vi "LDLTS measurement.vi"(5 "Session properties":T5, 7 "Workspace":path, 8 "Error In":errorcluster, 9 "myDLTS file path":path=path "", 10 "LDLTS measurement":T2={"Name"="", "Comment"="", "Time"=timestamp(0 s since 1904-01-01), "Folder"=path "", "LDLTS properties"={"T"=0.0, "Test signal"=0.0, "Test frequency"=0.0, "Bandwidth"=0.0, "Averaging"=0.0, "Vbias"=0.0, "Vpulse"=0.0, "pulse length"=0.0, "Pulse 2"=FALSE, "Vpulse 2"=0.0, "pulse length 2"=0.0, "I range"=-2.0, "V range"=10.0, "Sampling rate"=0.0, "Acq. delay"=0.0, "Sampling time"=0.0, "Filter order"=0, "Equivalent circuit model"=0}, "GUID"=""} {"LDLTS properties"."Equivalent circuit model" items=["Rp || Cp", "Rs + Cs", "Rs + Ls", "G B", "D Cs", "Q Cs", "D Ls", "Q Ls", "Rp || Lp", "D Cp"]; "LDLTS properties"."Filter order" min=0 max=8 step=1; "LDLTS properties"."Sampling rate" items=["13k"=13392.857422, "27k"=26785.714844, "54k"=53571.429687, "107k"=107142.859375]; "LDLTS properties"."V range" items=["10mV"=0.01, "100mV"=0.1, "1V"=1.0, "10V"=10.0]; "LDLTS properties"."I range" items=["100nA"=-7.0, "1µA"=-6.0, "10µA"=-5.0, "100µA"=-4.0, "1mA"=-3.0, "10mA"=-2.0]}, 11 "Loop data":T6={"Persistent"={"Last file"=path "", "Last user"="", "Users"=[]}, "Temp handle"={"Connected"=FALSE, "Temp ctrl"={"Gain (P)"=0.0, "Reset (I)"=0.0, "Rate (D)"=0.0, "Stabilization rate"=0.0, "Stabilization delta"=0.0, "Type"=enum."Lake Shore 325", "Custom temp ctrl"={"VISA resource name"=""}, "Lakeshore 325"={"VISA name"="", "Loop"=0, "Heater Range"=1, "Heater Resistance"=0, "Sample sensor"=0, "Fast sensor"=0, "Slow sensor"=0}, "Lakeshore 331"={"VISA name"="", "Loop"=1, "Heater Range"=0, "Sample sensor"=0, "Fast sensor"=0, "Slow sensor"=0}, "Lakeshore 332"={"VISA name"="", "Loop"=1, "Heater Range"=0, "Sample sensor"=0, "Fast sensor"=0, "Slow sensor"=0}, "Lakeshore 335"={"VISA name"="", "Loop"=1, "Sample sensor"=0, "Fast sensor"=0, "Slow sensor"=0, "Heater Range"=0, "Output mode"=enum."Off"}, "Lakeshore 336"={"VISA name"="", "Loop"=1, "Output mode"=enum."Off", "Max current"=1.0, "Heater resistance"=1, "Sample sensor"=1, "Slow sensor"=1, "Fast sensor"=1}}}, "Paths"={"Manual"=path "", "Settings"=path "", "Persistent"=path "", "Work dir."=path ""}, "Settings"={"MFIA"={"Address"="", "Use compensation"=TRUE, "Shut down gracefully"=FALSE}, "Temp ctrl"={"Gain (P)"=0.0, "Reset (I)"=0.0, "Rate (D)"=0.0, "Stabilization rate"=0.0, "Stabilization delta"=0.0, "Type"=enum."Lake Shore 325", "Custom temp ctrl"={"VISA resource name"=""}, "Lakeshore 325"={"VISA name"="", "Loop"=0, "Heater Range"=1, "Heater Resistance"=0, "Sample sensor"=0, "Fast sensor"=0, "Slow sensor"=0}, "Lakeshore 331"={"VISA name"="", "Loop"=1, "Heater Range"=0, "Sample sensor"=0, "Fast sensor"=0, "Slow sensor"=0}, "Lakeshore 332"={"VISA name"="", "Loop"=1, "Heater Range"=0, "Sample sensor"=0, "Fast sensor"=0, "Slow sensor"=0}, "Lakeshore 335"={"VISA name"="", "Loop"=1, "Sample sensor"=0, "Fast sensor"=0, "Slow sensor"=0, "Heater Range"=0, "Output mode"=enum."Off"}, "Lakeshore 336"={"VISA name"="", "Loop"=1, "Output mode"=enum."Off", "Max current"=1.0, "Heater resistance"=1, "Sample sensor"=1, "Slow sensor"=1, "Fast sensor"=1}}, "Source-meter"={"Type"=enum."Custom", "Custom source-meter"={"VISA resource name"=""}, "Keithley 2600"={"VISA name"="", "Ignore ID Query"=FALSE, "SMU"=enum."Channel A"}, "Keithley 2400 Series"={"VISA name"="", "Ignore ID Query"=FALSE}}, "Other"={"Enable OriginLab"=FALSE, "Reader mode"=FALSE, "Auto-save"=FALSE}, "Defaults"={"IV properties"={"T"=0.0, "Vstart"=-0.5, "Vstop"=0.5, "Vpoints"=10.0, "Settling"=0.01, "I limit"=0.1, "Log mapping"=FALSE, "Averaging"=0.0}, "CV properties"={"T"=0.0, "Vstart"=-0.5, "Vstop"=0.5, "Vpoints"=10.0, "Precision"=enum."Normal", "Test signal"=0.01, "Auto I range"=FALSE, "Test frequency"=100000.0, "I range"=-2.0, "V range"=10.0, "Log mapping"=FALSE, "Rel perm"=0.0, "Area"=0.0, "Equivalent circuit model"=0}, "DLTS properties"={"Tstart"=0.0, "Instant start"=FALSE, "Tstop"=0.0, "T rate"=0.0, "Test signal"=0.0, "Test frequency"=0.0, "Bandwidth"=0.0, "Averaging"=0.0, "Vbias"=0.0, "Vpulse"=0.0, "pulse length"=0.0, "Pulse 2"=FALSE, "Vpulse 2"=0.0, "pulse length 2"=0.0, "I range"=-2.0, "V range"=10.0, "Emission rate"=[], "Sampling rate"=0.0, "Acq. delay"=0.0, "Filter order"=0, "Equivalent circuit model"=0}, "LDLTS properties"={"T"=0.0, "Test signal"=0.0, "Test frequency"=0.0, "Bandwidth"=0.0, "Averaging"=0.0, "Vbias"=0.0, "Vpulse"=0.0, "pulse length"=0.0, "Pulse 2"=FALSE, "Vpulse 2"=0.0, "pulse length 2"=0.0, "I range"=-2.0, "V range"=10.0, "Sampling rate"=0.0, "Acq. delay"=0.0, "Sampling time"=0.0, "Filter order"=0, "Equivalent circuit model"=0}}}, "Software version"=0.0, "MFIA handle"={"ziHandle"={"handleValid"=FALSE, "Conn"=0, "Path Prefix"="", "Handle"=0, "Connected"=FALSE, "Clockbase(s)"=0.0}, "Selected device"="", "ziModHandle"={"handleValid"=FALSE, "Conn"=0, "ModHandle"=0, "moduleID"="", "Path Prefix"=""}}, "Source-meter handle"={"Connected"=FALSE, "Source-meter"={"Type"=enum."Custom", "Custom source-meter"={"VISA resource name"=""}, "Keithley 2600"={"VISA name"="", "Ignore ID Query"=FALSE, "SMU"=enum."Channel A"}, "Keithley 2400 Series"={"VISA name"="", "Ignore ID Query"=FALSE}}}} {"MFIA handle"."ziModHandle"."ModHandle" format="0x%08x"; "MFIA handle"."ziModHandle"."Conn" format="0x%08x"; "MFIA handle"."ziHandle"."Handle" format="0x%08x"; "MFIA handle"."ziHandle"."Conn" format="0x%08x"; "Settings"."Defaults"."LDLTS properties"."Equivalent circuit model" items=["Rp || Cp", "Rs + Cs", "Rs + Ls", "G B", "D Cs", "Q Cs", "D Ls", "Q Ls", "Rp || Lp", "D Cp"]; "Settings"."Defaults"."LDLTS properties"."Filter order" min=0 max=8 step=1; "Settings"."Defaults"."LDLTS properties"."Sampling rate" items=["13k"=13392.857422, "27k"=26785.714844, "54k"=53571.429687, "107k"=107142.859375]; "Settings"."Defaults"."LDLTS properties"."V range" items=["10mV"=0.01, "100mV"=0.1, "1V"=1.0, "10V"=10.0]; "Settings"."Defaults"."LDLTS properties"."I range" items=["100nA"=-7.0, "1µA"=-6.0, "10µA"=-5.0, "100µA"=-4.0, "1mA"=-3.0, "10mA"=-2.0]; "Settings"."Defaults"."DLTS properties"."Equivalent circuit model" items=["Rp || Cp", "Rs + Cs", "Rs + Ls", "G B", "D Cs", "Q Cs", "D Ls", "Q Ls", "Rp || Lp", "D Cp"]; "Settings"."Defaults"."DLTS properties"."Filter order" min=0 max=8 step=1; "Settings"."Defaults"."DLTS properties"."Sampling rate" items=["13k"=13392.857422, "27k"=26785.714844, "54k"=53571.429687, "107k"=107142.859375]; "Settings"."Defaults"."DLTS properties"."V range" items=["10mV"=0.01, "100mV"=0.1, "1V"=1.0, "10V"=10.0]; "Settings"."Defaults"."DLTS properties"."I range" items=["10mV"=0.01, "100mV"=0.1, "1V"=1.0, "10V"=10.0]; "Settings"."Defaults"."CV properties"."Equivalent circuit model" items=["Rp || Cp", "Rs + Cs", "Rs + Ls", "G B", "D Cs", "Q Cs", "D Ls", "Q Ls", "Rp || Lp", "D Cp"]; "Settings"."Defaults"."CV properties"."V range" items=["10mV"=0.01, "100mV"=0.1, "1V"=1.0, "10V"=10.0]; "Settings"."Defaults"."CV properties"."I range" items=["100nA"=-7.0, "1µA"=-6.0, "10µA"=-5.0, "100µA"=-4.0, "1mA"=-3.0, "10mA"=-2.0]; "Settings"."Defaults"."IV properties"."Settling" min=0.0 max=65535.0; "Settings"."Temp ctrl"."Lakeshore 336"."Fast sensor" items=["Sensor A", "Sensor B", "Sensor C", "Sensor D"]; "Settings"."Temp ctrl"."Lakeshore 336"."Slow sensor" items=["Sensor A", "Sensor B", "Sensor C", "Sensor D"]; "Settings"."Temp ctrl"."Lakeshore 336"."Sample sensor" items=["Sensor A", "Sensor B", "Sensor C", "Sensor D"]; "Settings"."Temp ctrl"."Lakeshore 336"."Heater resistance" items=["25 Ohm"=1, "50 Ohm"=2]; "Settings"."Temp ctrl"."Lakeshore 336"."Max current" items=["0.707 A"=0.0, "1 A"=1.0, "1.414 A"=1.414, "2 A"=2.0]; "Settings"."Temp ctrl"."Lakeshore 336"."Loop" items=["Output 1"=1, "Output 2"=2, "Output 3"=3, "Output 4"=4]; "Settings"."Temp ctrl"."Lakeshore 335"."Heater Range" items=["Off", "Low (On)", "Medium", "High"]; "Settings"."Temp ctrl"."Lakeshore 335"."Slow sensor" items=["A", "B"]; "Settings"."Temp ctrl"."Lakeshore 335"."Fast sensor" items=["A", "B"]; "Settings"."Temp ctrl"."Lakeshore 335"."Sample sensor" items=["A", "B"]; "Settings"."Temp ctrl"."Lakeshore 335"."Loop" items=["Loop 1"=1, "Loop 2"=2]; "Settings"."Temp ctrl"."Lakeshore 332"."Slow sensor" items=["A", "B"]; "Settings"."Temp ctrl"."Lakeshore 332"."Fast sensor" items=["A", "B"]; "Settings"."Temp ctrl"."Lakeshore 332"."Sample sensor" items=["A", "B"]; "Settings"."Temp ctrl"."Lakeshore 332"."Heater Range" items=["Off", "Low (0.5W)", "Med (5W)", "High (50W)"]; "Settings"."Temp ctrl"."Lakeshore 332"."Loop" items=["Loop 1", "Loop 2"]; "Settings"."Temp ctrl"."Lakeshore 331"."Slow sensor" items=["A", "B"]; "Settings"."Temp ctrl"."Lakeshore 331"."Fast sensor" items=["A", "B"]; "Settings"."Temp ctrl"."Lakeshore 331"."Sample sensor" items=["A", "B"]; "Settings"."Temp ctrl"."Lakeshore 331"."Heater Range" items=["Off", "Low (0.5W)", "Med (5W)", "High (50W)"]; "Settings"."Temp ctrl"."Lakeshore 331"."Loop" items=["Loop 1", "Loop 2"]; "Settings"."Temp ctrl"."Lakeshore 325"."Slow sensor" items=["A", "B"]; "Settings"."Temp ctrl"."Lakeshore 325"."Fast sensor" items=["A", "B"]; "Settings"."Temp ctrl"."Lakeshore 325"."Sample sensor" items=["A", "B"]; "Settings"."Temp ctrl"."Lakeshore 325"."Heater Resistance" items=["25 Ohm"=1, "50 Ohm"=2]; "Settings"."Temp ctrl"."Lakeshore 325"."Heater Range" items=["Off", "Low (loop 1) or On (loop 2)", "High (loop 1)"]; "Settings"."Temp ctrl"."Lakeshore 325"."Loop" items=["Loop 1"=1, "Loop 2"=2]; "Temp handle"."Temp ctrl"."Lakeshore 336"."Fast sensor" items=["Sensor A", "Sensor B", "Sensor C", "Sensor D"]; "Temp handle"."Temp ctrl"."Lakeshore 336"."Slow sensor" items=["Sensor A", "Sensor B", "Sensor C", "Sensor D"]; "Temp handle"."Temp ctrl"."Lakeshore 336"."Sample sensor" items=["Sensor A", "Sensor B", "Sensor C", "Sensor D"]; "Temp handle"."Temp ctrl"."Lakeshore 336"."Heater resistance" items=["25 Ohm"=1, "50 Ohm"=2]; "Temp handle"."Temp ctrl"."Lakeshore 336"."Max current" items=["0.707 A"=0.0, "1 A"=1.0, "1.414 A"=1.414, "2 A"=2.0]; "Temp handle"."Temp ctrl"."Lakeshore 336"."Loop" items=["Output 1"=1, "Output 2"=2, "Output 3"=3, "Output 4"=4]; "Temp handle"."Temp ctrl"."Lakeshore 335"."Heater Range" items=["Off", "Low (On)", "Medium", "High"]; "Temp handle"."Temp ctrl"."Lakeshore 335"."Slow sensor" items=["A", "B"]; "Temp handle"."Temp ctrl"."Lakeshore 335"."Fast sensor" items=["A", "B"]; "Temp handle"."Temp ctrl"."Lakeshore 335"."Sample sensor" items=["A", "B"]; "Temp handle"."Temp ctrl"."Lakeshore 335"."Loop" items=["Loop 1"=1, "Loop 2"=2]; "Temp handle"."Temp ctrl"."Lakeshore 332"."Slow sensor" items=["A", "B"]; "Temp handle"."Temp ctrl"."Lakeshore 332"."Fast sensor" items=["A", "B"]; "Temp handle"."Temp ctrl"."Lakeshore 332"."Sample sensor" items=["A", "B"]; "Temp handle"."Temp ctrl"."Lakeshore 332"."Heater Range" items=["Off", "Low (0.5W)", "Med (5W)", "High (50W)"]; "Temp handle"."Temp ctrl"."Lakeshore 332"."Loop" items=["Loop 1", "Loop 2"]; "Temp handle"."Temp ctrl"."Lakeshore 331"."Slow sensor" items=["A", "B"]; "Temp handle"."Temp ctrl"."Lakeshore 331"."Fast sensor" items=["A", "B"]; "Temp handle"."Temp ctrl"."Lakeshore 331"."Sample sensor" items=["A", "B"]; "Temp handle"."Temp ctrl"."Lakeshore 331"."Heater Range" items=["Off", "Low (0.5W)", "Med (5W)", "High (50W)"]; "Temp handle"."Temp ctrl"."Lakeshore 331"."Loop" items=["Loop 1", "Loop 2"]; "Temp handle"."Temp ctrl"."Lakeshore 325"."Slow sensor" items=["A", "B"]; "Temp handle"."Temp ctrl"."Lakeshore 325"."Fast sensor" items=["A", "B"]; "Temp handle"."Temp ctrl"."Lakeshore 325"."Sample sensor" items=["A", "B"]; "Temp handle"."Temp ctrl"."Lakeshore 325"."Heater Resistance" items=["25 Ohm"=1, "50 Ohm"=2]; "Temp handle"."Temp ctrl"."Lakeshore 325"."Heater Range" items=["Off", "Low (loop 1) or On (loop 2)", "High (loop 1)"]; "Temp handle"."Temp ctrl"."Lakeshore 325"."Loop" items=["Loop 1"=1, "Loop 2"=2]}) -> (0 "Error Out":errorcluster, 1 "Modified":bool, 2 "LDLTS measurement out":T2={"Name"="", "Comment"="", "Time"=timestamp(0 s since 1904-01-01), "Folder"=path "", "LDLTS properties"={"T"=0.0, "Test signal"=0.0, "Test frequency"=0.0, "Bandwidth"=0.0, "Averaging"=0.0, "Vbias"=0.0, "Vpulse"=0.0, "pulse length"=0.0, "Pulse 2"=FALSE, "Vpulse 2"=0.0, "pulse length 2"=0.0, "I range"=-2.0, "V range"=10.0, "Sampling rate"=0.0, "Acq. delay"=0.0, "Sampling time"=0.0, "Filter order"=0, "Equivalent circuit model"=0}, "GUID"=""} {"LDLTS properties"."Equivalent circuit model" items=["Rp || Cp", "Rs + Cs", "Rs + Ls", "G B", "D Cs", "Q Cs", "D Ls", "Q Ls", "Rp || Lp", "D Cp"]; "LDLTS properties"."Filter order" min=0 max=8 step=1; "LDLTS properties"."Sampling rate" items=["13k"=13392.857422, "27k"=26785.714844, "54k"=53571.429687, "107k"=107142.859375]; "LDLTS properties"."V range" items=["10mV"=0.01, "100mV"=0.1, "1V"=1.0, "10V"=10.0]; "LDLTS properties"."I range" items=["100nA"=-7.0, "1µA"=-6.0, "10µA"=-5.0, "100µA"=-4.0, "1mA"=-3.0, "10mA"=-2.0]}, 3 "Loop data out":T6={"Persistent"={"Last file"=path "", "Last user"="", "Users"=[]}, "Temp handle"={"Connected"=FALSE, "Temp ctrl"={"Gain (P)"=0.0, "Reset (I)"=0.0, "Rate (D)"=0.0, "Stabilization rate"=0.0, "Stabilization delta"=0.0, "Type"=enum."Lake Shore 325", "Custom temp ctrl"={"VISA resource name"=""}, "Lakeshore 325"={"VISA name"="", "Loop"=0, "Heater Range"=1, "Heater Resistance"=0, "Sample sensor"=0, "Fast sensor"=0, "Slow sensor"=0}, "Lakeshore 331"={"VISA name"="", "Loop"=1, "Heater Range"=0, "Sample sensor"=0, "Fast sensor"=0, "Slow sensor"=0}, "Lakeshore 332"={"VISA name"="", "Loop"=1, "Heater Range"=0, "Sample sensor"=0, "Fast sensor"=0, "Slow sensor"=0}, "Lakeshore 335"={"VISA name"="", "Loop"=1, "Sample sensor"=0, "Fast sensor"=0, "Slow sensor"=0, "Heater Range"=0, "Output mode"=enum."Off"}, "Lakeshore 336"={"VISA name"="", "Loop"=1, "Output mode"=enum."Off", "Max current"=1.0, "Heater resistance"=1, "Sample sensor"=1, "Slow sensor"=1, "Fast sensor"=1}}}, "Paths"={"Manual"=path "", "Settings"=path "", "Persistent"=path "", "Work dir."=path ""}, "Settings"={"MFIA"={"Address"="", "Use compensation"=TRUE, "Shut down gracefully"=FALSE}, "Temp ctrl"={"Gain (P)"=0.0, "Reset (I)"=0.0, "Rate (D)"=0.0, "Stabilization rate"=0.0, "Stabilization delta"=0.0, "Type"=enum."Lake Shore 325", "Custom temp ctrl"={"VISA resource name"=""}, "Lakeshore 325"={"VISA name"="", "Loop"=0, "Heater Range"=1, "Heater Resistance"=0, "Sample sensor"=0, "Fast sensor"=0, "Slow sensor"=0}, "Lakeshore 331"={"VISA name"="", "Loop"=1, "Heater Range"=0, "Sample sensor"=0, "Fast sensor"=0, "Slow sensor"=0}, "Lakeshore 332"={"VISA name"="", "Loop"=1, "Heater Range"=0, "Sample sensor"=0, "Fast sensor"=0, "Slow sensor"=0}, "Lakeshore 335"={"VISA name"="", "Loop"=1, "Sample sensor"=0, "Fast sensor"=0, "Slow sensor"=0, "Heater Range"=0, "Output mode"=enum."Off"}, "Lakeshore 336"={"VISA name"="", "Loop"=1, "Output mode"=enum."Off", "Max current"=1.0, "Heater resistance"=1, "Sample sensor"=1, "Slow sensor"=1, "Fast sensor"=1}}, "Source-meter"={"Type"=enum."Custom", "Custom source-meter"={"VISA resource name"=""}, "Keithley 2600"={"VISA name"="", "Ignore ID Query"=FALSE, "SMU"=enum."Channel A"}, "Keithley 2400 Series"={"VISA name"="", "Ignore ID Query"=FALSE}}, "Other"={"Enable OriginLab"=FALSE, "Reader mode"=FALSE, "Auto-save"=FALSE}, "Defaults"={"IV properties"={"T"=0.0, "Vstart"=-0.5, "Vstop"=0.5, "Vpoints"=10.0, "Settling"=0.01, "I limit"=0.1, "Log mapping"=FALSE, "Averaging"=0.0}, "CV properties"={"T"=0.0, "Vstart"=-0.5, "Vstop"=0.5, "Vpoints"=10.0, "Precision"=enum."Normal", "Test signal"=0.01, "Auto I range"=FALSE, "Test frequency"=100000.0, "I range"=-2.0, "V range"=10.0, "Log mapping"=FALSE, "Rel perm"=0.0, "Area"=0.0, "Equivalent circuit model"=0}, "DLTS properties"={"Tstart"=0.0, "Instant start"=FALSE, "Tstop"=0.0, "T rate"=0.0, "Test signal"=0.0, "Test frequency"=0.0, "Bandwidth"=0.0, "Averaging"=0.0, "Vbias"=0.0, "Vpulse"=0.0, "pulse length"=0.0, "Pulse 2"=FALSE, "Vpulse 2"=0.0, "pulse length 2"=0.0, "I range"=-2.0, "V range"=10.0, "Emission rate"=[], "Sampling rate"=0.0, "Acq. delay"=0.0, "Filter order"=0, "Equivalent circuit model"=0}, "LDLTS properties"={"T"=0.0, "Test signal"=0.0, "Test frequency"=0.0, "Bandwidth"=0.0, "Averaging"=0.0, "Vbias"=0.0, "Vpulse"=0.0, "pulse length"=0.0, "Pulse 2"=FALSE, "Vpulse 2"=0.0, "pulse length 2"=0.0, "I range"=-2.0, "V range"=10.0, "Sampling rate"=0.0, "Acq. delay"=0.0, "Sampling time"=0.0, "Filter order"=0, "Equivalent circuit model"=0}}}, "Software version"=0.0, "MFIA handle"={"ziHandle"={"handleValid"=FALSE, "Conn"=0, "Path Prefix"="", "Handle"=0, "Connected"=FALSE, "Clockbase(s)"=0.0}, "Selected device"="", "ziModHandle"={"handleValid"=FALSE, "Conn"=0, "ModHandle"=0, "moduleID"="", "Path Prefix"=""}}, "Source-meter handle"={"Connected"=FALSE, "Source-meter"={"Type"=enum."Custom", "Custom source-meter"={"VISA resource name"=""}, "Keithley 2600"={"VISA name"="", "Ignore ID Query"=FALSE, "SMU"=enum."Channel A"}, "Keithley 2400 Series"={"VISA name"="", "Ignore ID Query"=FALSE}}}} {"MFIA handle"."ziModHandle"."ModHandle" format="0x%08x"; "MFIA handle"."ziModHandle"."Conn" format="0x%08x"; "MFIA handle"."ziHandle"."Handle" format="0x%08x"; "MFIA handle"."ziHandle"."Conn" format="0x%08x"; "Settings"."Defaults"."LDLTS properties"."Equivalent circuit model" items=["Rp || Cp", "Rs + Cs", "Rs + Ls", "G B", "D Cs", "Q Cs", "D Ls", "Q Ls", "Rp || Lp", "D Cp"]; "Settings"."Defaults"."LDLTS properties"."Filter order" min=0 max=8 step=1; "Settings"."Defaults"."LDLTS properties"."Sampling rate" items=["13k"=13392.857422, "27k"=26785.714844, "54k"=53571.429687, "107k"=107142.859375]; "Settings"."Defaults"."LDLTS properties"."V range" items=["10mV"=0.01, "100mV"=0.1, "1V"=1.0, "10V"=10.0]; "Settings"."Defaults"."LDLTS properties"."I range" items=["100nA"=-7.0, "1µA"=-6.0, "10µA"=-5.0, "100µA"=-4.0, "1mA"=-3.0, "10mA"=-2.0]; "Settings"."Defaults"."DLTS properties"."Equivalent circuit model" items=["Rp || Cp", "Rs + Cs", "Rs + Ls", "G B", "D Cs", "Q Cs", "D Ls", "Q Ls", "Rp || Lp", "D Cp"]; "Settings"."Defaults"."DLTS properties"."Filter order" min=0 max=8 step=1; "Settings"."Defaults"."DLTS properties"."Sampling rate" items=["13k"=13392.857422, "27k"=26785.714844, "54k"=53571.429687, "107k"=107142.859375]; "Settings"."Defaults"."DLTS properties"."V range" items=["10mV"=0.01, "100mV"=0.1, "1V"=1.0, "10V"=10.0]; "Settings"."Defaults"."DLTS properties"."I range" items=["10mV"=0.01, "100mV"=0.1, "1V"=1.0, "10V"=10.0]; "Settings"."Defaults"."CV properties"."Equivalent circuit model" items=["Rp || Cp", "Rs + Cs", "Rs + Ls", "G B", "D Cs", "Q Cs", "D Ls", "Q Ls", "Rp || Lp", "D Cp"]; "Settings"."Defaults"."CV properties"."V range" items=["10mV"=0.01, "100mV"=0.1, "1V"=1.0, "10V"=10.0]; "Settings"."Defaults"."CV properties"."I range" items=["100nA"=-7.0, "1µA"=-6.0, "10µA"=-5.0, "100µA"=-4.0, "1mA"=-3.0, "10mA"=-2.0]; "Settings"."Defaults"."IV properties"."Settling" min=0.0 max=65535.0; "Settings"."Temp ctrl"."Lakeshore 336"."Fast sensor" items=["Sensor A", "Sensor B", "Sensor C", "Sensor D"]; "Settings"."Temp ctrl"."Lakeshore 336"."Slow sensor" items=["Sensor A", "Sensor B", "Sensor C", "Sensor D"]; "Settings"."Temp ctrl"."Lakeshore 336"."Sample sensor" items=["Sensor A", "Sensor B", "Sensor C", "Sensor D"]; "Settings"."Temp ctrl"."Lakeshore 336"."Heater resistance" items=["25 Ohm"=1, "50 Ohm"=2]; "Settings"."Temp ctrl"."Lakeshore 336"."Max current" items=["0.707 A"=0.0, "1 A"=1.0, "1.414 A"=1.414, "2 A"=2.0]; "Settings"."Temp ctrl"."Lakeshore 336"."Loop" items=["Output 1"=1, "Output 2"=2, "Output 3"=3, "Output 4"=4]; "Settings"."Temp ctrl"."Lakeshore 335"."Heater Range" items=["Off", "Low (On)", "Medium", "High"]; "Settings"."Temp ctrl"."Lakeshore 335"."Slow sensor" items=["A", "B"]; "Settings"."Temp ctrl"."Lakeshore 335"."Fast sensor" items=["A", "B"]; "Settings"."Temp ctrl"."Lakeshore 335"."Sample sensor" items=["A", "B"]; "Settings"."Temp ctrl"."Lakeshore 335"."Loop" items=["Loop 1"=1, "Loop 2"=2]; "Settings"."Temp ctrl"."Lakeshore 332"."Slow sensor" items=["A", "B"]; "Settings"."Temp ctrl"."Lakeshore 332"."Fast sensor" items=["A", "B"]; "Settings"."Temp ctrl"."Lakeshore 332"."Sample sensor" items=["A", "B"]; "Settings"."Temp ctrl"."Lakeshore 332"."Heater Range" items=["Off", "Low (0.5W)", "Med (5W)", "High (50W)"]; "Settings"."Temp ctrl"."Lakeshore 332"."Loop" items=["Loop 1", "Loop 2"]; "Settings"."Temp ctrl"."Lakeshore 331"."Slow sensor" items=["A", "B"]; "Settings"."Temp ctrl"."Lakeshore 331"."Fast sensor" items=["A", "B"]; "Settings"."Temp ctrl"."Lakeshore 331"."Sample sensor" items=["A", "B"]; "Settings"."Temp ctrl"."Lakeshore 331"."Heater Range" items=["Off", "Low (0.5W)", "Med (5W)", "High (50W)"]; "Settings"."Temp ctrl"."Lakeshore 331"."Loop" items=["Loop 1", "Loop 2"]; "Settings"."Temp ctrl"."Lakeshore 325"."Slow sensor" items=["A", "B"]; "Settings"."Temp ctrl"."Lakeshore 325"."Fast sensor" items=["A", "B"]; "Settings"."Temp ctrl"."Lakeshore 325"."Sample sensor" items=["A", "B"]; "Settings"."Temp ctrl"."Lakeshore 325"."Heater Resistance" items=["25 Ohm"=1, "50 Ohm"=2]; "Settings"."Temp ctrl"."Lakeshore 325"."Heater Range" items=["Off", "Low (loop 1) or On (loop 2)", "High (loop 1)"]; "Settings"."Temp ctrl"."Lakeshore 325"."Loop" items=["Loop 1"=1, "Loop 2"=2]; "Temp handle"."Temp ctrl"."Lakeshore 336"."Fast sensor" items=["Sensor A", "Sensor B", "Sensor C", "Sensor D"]; "Temp handle"."Temp ctrl"."Lakeshore 336"."Slow sensor" items=["Sensor A", "Sensor B", "Sensor C", "Sensor D"]; "Temp handle"."Temp ctrl"."Lakeshore 336"."Sample sensor" items=["Sensor A", "Sensor B", "Sensor C", "Sensor D"]; "Temp handle"."Temp ctrl"."Lakeshore 336"."Heater resistance" items=["25 Ohm"=1, "50 Ohm"=2]; "Temp handle"."Temp ctrl"."Lakeshore 336"."Max current" items=["0.707 A"=0.0, "1 A"=1.0, "1.414 A"=1.414, "2 A"=2.0]; "Temp handle"."Temp ctrl"."Lakeshore 336"."Loop" items=["Output 1"=1, "Output 2"=2, "Output 3"=3, "Output 4"=4]; "Temp handle"."Temp ctrl"."Lakeshore 335"."Heater Range" items=["Off", "Low (On)", "Medium", "High"]; "Temp handle"."Temp ctrl"."Lakeshore 335"."Slow sensor" items=["A", "B"]; "Temp handle"."Temp ctrl"."Lakeshore 335"."Fast sensor" items=["A", "B"]; "Temp handle"."Temp ctrl"."Lakeshore 335"."Sample sensor" items=["A", "B"]; "Temp handle"."Temp ctrl"."Lakeshore 335"."Loop" items=["Loop 1"=1, "Loop 2"=2]; "Temp handle"."Temp ctrl"."Lakeshore 332"."Slow sensor" items=["A", "B"]; "Temp handle"."Temp ctrl"."Lakeshore 332"."Fast sensor" items=["A", "B"]; "Temp handle"."Temp ctrl"."Lakeshore 332"."Sample sensor" items=["A", "B"]; "Temp handle"."Temp ctrl"."Lakeshore 332"."Heater Range" items=["Off", "Low (0.5W)", "Med (5W)", "High (50W)"]; "Temp handle"."Temp ctrl"."Lakeshore 332"."Loop" items=["Loop 1", "Loop 2"]; "Temp handle"."Temp ctrl"."Lakeshore 331"."Slow sensor" items=["A", "B"]; "Temp handle"."Temp ctrl"."Lakeshore 331"."Fast sensor" items=["A", "B"]; "Temp handle"."Temp ctrl"."Lakeshore 331"."Sample sensor" items=["A", "B"]; "Temp handle"."Temp ctrl"."Lakeshore 331"."Heater Range" items=["Off", "Low (0.5W)", "Med (5W)", "High (50W)"]; "Temp handle"."Temp ctrl"."Lakeshore 331"."Loop" items=["Loop 1", "Loop 2"]; "Temp handle"."Temp ctrl"."Lakeshore 325"."Slow sensor" items=["A", "B"]; "Temp handle"."Temp ctrl"."Lakeshore 325"."Fast sensor" items=["A", "B"]; "Temp handle"."Temp ctrl"."Lakeshore 325"."Sample sensor" items=["A", "B"]; "Temp handle"."Temp ctrl"."Lakeshore 325"."Heater Resistance" items=["25 Ohm"=1, "50 Ohm"=2]; "Temp handle"."Temp ctrl"."Lakeshore 325"."Heater Range" items=["Off", "Low (loop 1) or On (loop 2)", "High (loop 1)"]; "Temp handle"."Temp ctrl"."Lakeshore 325"."Loop" items=["Loop 1"=1, "Loop 2"=2]})   [LabVIEW 2019]
doc: "Handles LDLTS measurement, displays LDLTS GUI window"
uses:
  Type defs/Loop data Type Def.ctl
  Type defs/Persistent Type Def.ctl
  Type defs/Temp handle Type Def.ctl
  Type defs/Temp ctrl Type Def.ctl
  Custom devices/Custom temp ctrl settings.ctl
  Type defs/Paths Type Def.ctl
  Type defs/Settings Type Def.ctl
  Type defs/Imps Type Def.ctl
  Type defs/Source-meter Type Def.ctl
  Custom devices/Custom source-meter settings.ctl
  Type defs/Other settings Type Def.ctl
  Type defs/IV properties Type Def.ctl
  Type defs/CV properties Type Def.ctl
  Type defs/DLTS properties Type Def.ctl
  Type defs/LDLTS properties Type Def.ctl
  Type defs/MFIA handle Type Def.ctl
  <instrlib>/Zurich Instruments LabOne/Public/ziTypeHandle.ctl
  <instrlib>/Zurich Instruments LabOne/Public/Modules/ziTypeModHandle.ctl
  Type defs/Source-meter handle Type Def.ctl
  Type defs/Session properties Type Def.ctl
  Type defs/LDLTS measurement Type Def.ctl
  <vilib>/Utility/miscctls.llb/LVPointTypeDef.ctl
  <vilib>/Utility/error.llb/DialogType.ctl
  <vilib>/TaskbarProgressAPI/_TypeDefs/Progress State.ctl
  Export single clipboard - LDLTS cluster.vi
  Export single dat - LDLTS cluster.vi
  Export Origin - LDLTS.vi
  <vilib>/TaskbarProgressAPI/TaskbarProgressAPI.lvlib
  <instrlib>/Zurich Instruments LabOne/Zurich Instruments LabOne.lvlib
panel:
  in  "Voltage remove":T1(ring) caption="Enum"
  in  "Model":u16(ring) caption="Equivalent circuit model" items=["Rp || Cp", "Rs + Cs"]
  in  "Filter order":i32=8 caption="Numeric" min=1 max=8 step=1
  out "Filter rise time":dbl[unit]=10.0 caption="Numeric" min=0.1 max=100.0 format="%#_2p"
  in  "Stop":bool
  in  "Folder":path
  in  "2 pulse mode":bool caption="2 pulse mode:"
  in  "2nd pulse length":dbl[unit]=100.0 caption="2nd pulse duration" min=2.333e-07 max=1.0 format="%#.1p"
  in  "2nd pulse voltage":dbl[unit]=0.01 caption="Numeric" min=-10.0 max=10.0 format="%#_6p"
  in  "Capture duration":dbl[unit]=1.0 caption="Numeric" min=0.0 max=1000.0 step=1e-06 format="%#_6p"
  in  "Acquisition delay":dbl[unit]=1.0 caption="Numeric" min=0.0 max=1.0 step=1e-06 format="%#_6p"
  in  "Sampling rate":dbl(ring)=107142.859375 caption="Ring" items=["13 kSa"=13392.857422, "27 kSa"=26785.714844, "54 kSa"=53571.429687, "107 kSa"=107142.859375]
  in  "Bandwidth":dbl[unit]=10000.0 caption="Numeric" min=100.0 max=100000.0 format="%#_6p"
  out "No samples":dbl caption="Number of samples per transient" format="%#.0f"
  in  "Averaging":dbl=1.0 caption="Numeric" min=1.0 max=5000.0 step=1.0
  in  "1st pulse length":dbl[unit]=100.0 caption="1st pulse duration" min=2.333e-07 max=1.0 format="%#.1p"
  in  "1st pulse voltage":dbl[unit]=0.01 caption="Numeric" min=-10.0 max=10.0 format="%#_6p"
  in  "Bias voltage":dbl[unit]=0.01 caption="Numeric" min=-10.0 max=10.0 format="%#_6p"
  in  "V range":dbl[unit](ring)=10.0 caption="Voltage range" items=["10mV"=0.01, "100mV"=0.1, "1V"=1.0, "10V"=10.0]
  in  "Test frequency":dbl[unit]=100000.0 caption="Numeric" min=10000.0 max=5000000000.0 format="%#_6p"
  in  "I range":dbl(ring)=-7.0 caption="Current range" items=["100nA"=-7.0, "1µA"=-6.0, "10µA"=-5.0, "100µA"=-4.0, "1mA"=-3.0, "10mA"=-2.0]
  in  "Measure":bool
  in  "Test signal":dbl[unit]=0.3 caption="Numeric" min=1e-06 max=1.0 format="%#_6p"
  in  "Setpoint":dbl[unit]=1.0 caption="Numeric" min=1.0 max=800.0
  out "Temperature":dbl[unit] caption="Numeric"
  out "Measurement info":string
  in  "Top Buttons":T4
  out "Transient Graph":cluster{"t":dbl[], "Samples":dbl[]}(graph)
  out "Temp Chart":dbl(graph)=189.08
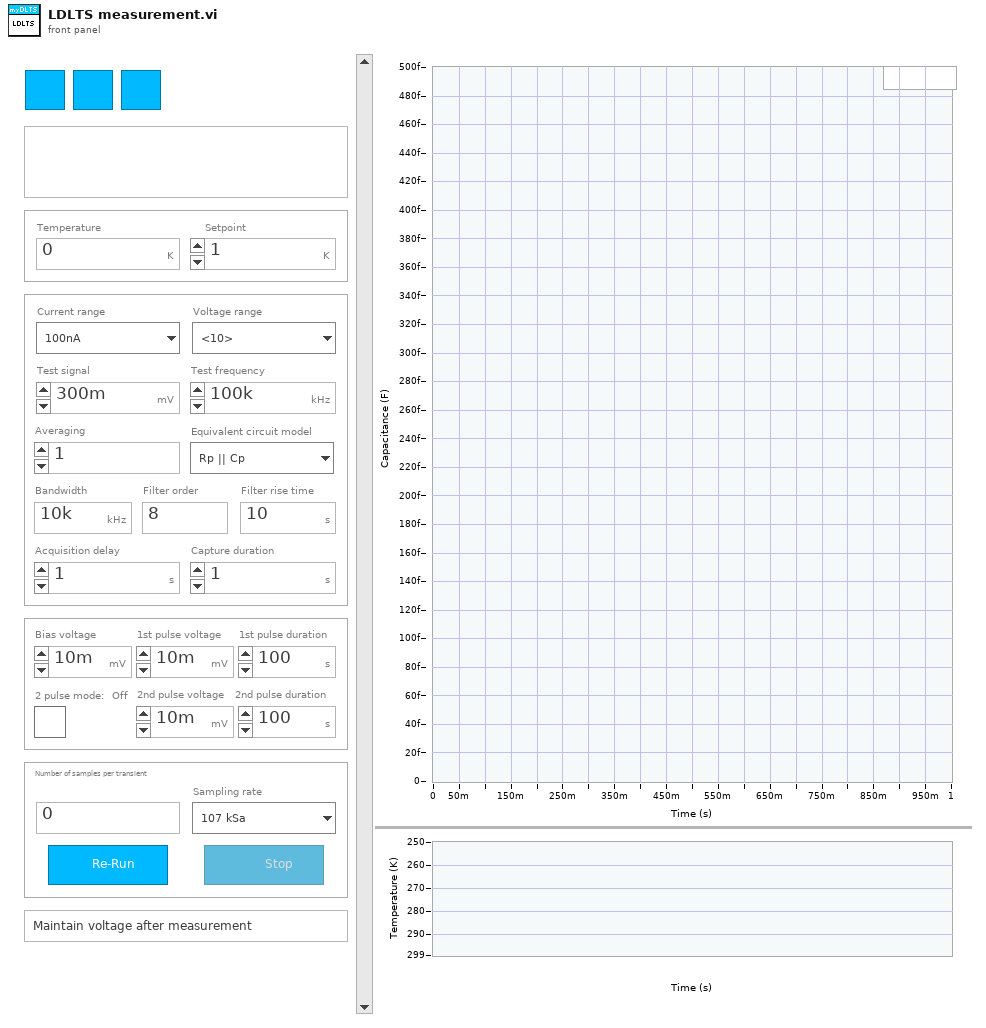
[diagram p1: front panel]
types:
  T1 = enum16{"Maintain voltage after measurement", "Disable voltage immediately after measurement"}
  T2 = typedef "LDLTS measurement Type Def.ctl" = cluster{"Name":string, "Comment":string, "Time":timestamp, "Folder":path, "LDLTS properties":T3, "GUID":string}
  T3 = typedef "LDLTS properties Type Def.ctl" = cluster{"T":dbl[unit], "Test signal":dbl[unit], "Test frequency":dbl[unit], "Bandwidth":dbl[unit], "Averaging":dbl, "Vbias":dbl[unit], "Vpulse":dbl[unit], "pulse length":dbl[unit], "Pulse 2":bool, "Vpulse 2":dbl[unit], "pulse length 2":dbl[unit], "I range":dbl, "V range":dbl[unit], "Sampling rate":dbl[unit], "Acq. delay":dbl[unit], "Sampling time":dbl[unit], "Filter order":i32, "Equivalent circuit model":u16}
  T4 = cluster{"Information":bool, "Help":bool, "Save Parameters":bool, "Export":bool}
  T5 = typedef "Session properties Type Def.ctl" = cluster{"Session name":string, "Comment":string, "User":string, "Software version":dbl, "Created":timestamp, "Modified":timestamp, "Binary":bool, "GUID":string}
  T6 = typedef "Loop data Type Def.ctl" = cluster{"Persistent":T7, "Temp handle":T8, "Paths":T11, "Settings":T12, "Software version":dbl, "MFIA handle":T20, "Source-meter handle":T23}
  T7 = typedef "Persistent Type Def.ctl" = cluster{"Last file":path, "Last user":string, "Users":cluster{"User":string, "Authors directory":path}[]}
  T8 = typedef "Temp handle Type Def.ctl" = cluster{"Connected":bool, "Temp ctrl":T9}
  T9 = typedef "Temp ctrl Type Def.ctl" = cluster{"Gain (P)":dbl, "Reset (I)":dbl, "Rate (D)":dbl, "Stabilization rate":dbl, "Stabilization delta":dbl, "Type":enum16{"Custom", "Lake Shore 325", "Lake Shore 331", "Lake Shore 332", "Lake Shore 335", "Lake Shore 336"}, "Custom temp ctrl":T10, "Lakeshore 325":cluster{"VISA name":refnum<visa-resource-name>, "Loop":u16, "Heater Range":u16, "Heater Resistance":u16, "Sample sensor":u16, "Fast sensor":u16, "Slow sensor":u16}, "Lakeshore 331":cluster{"VISA name":refnum<visa-resource-name>, "Loop":u16, "Heater Range":u16, "Sample sensor":u16, "Fast sensor":u16, "Slow sensor":u16}, "Lakeshore 332":cluster{"VISA name":refnum<visa-resource-name>, "Loop":u16, "Heater Range":u16, "Sample sensor":u16, "Fast sensor":u16, "Slow sensor":u16}, "Lakeshore 335":cluster{"VISA name":refnum<visa-resource-name>, "Loop":u16, "Sample sensor":u16, "Fast sensor":u16, "Slow sensor":u16, "Heater Range":u16, "Output mode":enum16{"Off", "Closed Loop PID", "Zone", "Open Loop", "Monitor Out", "Warmup Supply"}}, "Lakeshore 336":cluster{"VISA name":refnum<visa-resource-name>, "Loop":u16, "Output mode":enum16{"Off", "Closed Loop PID", "Zone", "Open Loop"}, "Max current":dbl, "Heater resistance":u16, "Sample sensor":u16, "Slow sensor":u16, "Fast sensor":u16}}
  T10 = typedef "Custom temp ctrl settings.ctl" = cluster{"VISA resource name":refnum<visa-resource-name>}
  T11 = typedef "Paths Type Def.ctl" = cluster{"Manual":path, "Settings":path, "Persistent":path, "Work dir.":path}
  T12 = typedef "Settings Type Def.ctl" = cluster{"MFIA":T13, "Temp ctrl":T9, "Source-meter":T14, "Other":T16, "Defaults":cluster{"IV properties":T17, "CV properties":T18, "DLTS properties":T19, "LDLTS properties":T3}}
  T13 = typedef "Imps Type Def.ctl" = cluster{"Address":string, "Use compensation":bool, "Shut down gracefully":bool}
  T14 = typedef "Source-meter Type Def.ctl" = cluster{"Type":enum16{"Custom", "Keithley 2600", "Keithley 2400 Series"}, "Custom source-meter":T15, "Keithley 2600":cluster{"VISA name":refnum<visa-resource-name>, "Ignore ID Query":bool, "SMU":enum16{"Channel A", "Channel B"}}, "Keithley 2400 Series":cluster{"VISA name":refnum<visa-resource-name>, "Ignore ID Query":bool}}
  T15 = typedef "Custom source-meter settings.ctl" = cluster{"VISA resource name":refnum<visa-resource-name>}
  T16 = typedef "Other settings Type Def.ctl" = cluster{"Enable OriginLab":bool, "Reader mode":bool, "Auto-save":bool}
  T17 = typedef "IV properties Type Def.ctl" = cluster{"T":dbl[unit], "Vstart":dbl[unit], "Vstop":dbl[unit], "Vpoints":dbl, "Settling":dbl[unit], "I limit":dbl[unit], "Log mapping":bool, "Averaging":dbl}
  T18 = typedef "CV properties Type Def.ctl" = cluster{"T":dbl[unit], "Vstart":dbl[unit], "Vstop":dbl[unit], "Vpoints":dbl, "Precision":enum16{"Low (Fast)", "Normal", "High (Slow)"}, "Test signal":dbl[unit], "Auto I range":bool, "Test frequency":dbl[unit], "I range":dbl, "V range":dbl[unit], "Log mapping":bool, "Rel perm":dbl, "Area":dbl[unit], "Equivalent circuit model":u16}
  T19 = typedef "DLTS properties Type Def.ctl" = cluster{"Tstart":dbl[unit], "Instant start":bool, "Tstop":dbl[unit], "T rate":dbl[unit], "Test signal":dbl[unit], "Test frequency":dbl[unit], "Bandwidth":dbl[unit], "Averaging":dbl, "Vbias":dbl[unit], "Vpulse":dbl[unit], "pulse length":dbl[unit], "Pulse 2":bool, "Vpulse 2":dbl[unit], "pulse length 2":dbl[unit], "I range":dbl, "V range":dbl[unit], "Emission rate":dbl[unit][], "Sampling rate":dbl[unit], "Acq. delay":dbl[unit], "Filter order":i32, "Equivalent circuit model":u16}
  T20 = typedef "MFIA handle Type Def.ctl" = cluster{"ziHandle":T21, "Selected device":string, "ziModHandle":T22}
  T21 = typedef "Zurich Instruments LabOne.lvlib/ziTypeHandle.ctl" = cluster{"handleValid":bool, "Conn":u64, "Path Prefix":string, "Handle":u64, "Connected":bool, "Clockbase(s)":dbl}
  T22 = typedef "Zurich Instruments LabOne.lvlib/ziTypeModHandle.ctl" = cluster{"handleValid":bool, "Conn":u64, "ModHandle":u64, "moduleID":string, "Path Prefix":string}
  T23 = typedef "Source-meter handle Type Def.ctl" = cluster{"Connected":bool, "Source-meter":T14}
  T24 = cluster{"MFIA":bool, "Temperature controller":bool, "Source meter":bool}
  T25 = typedef "LVPointTypeDef.ctl" = cluster{"Horizontal":i16, "Vertical":i16}
  T26 = enum8{"Enabled", "Disabled", "Disabled and Grayed Out"}
  T27 = typedef "Semaphore RefNum" = refnum<k1>
  T28 = typedef "DialogType.ctl" = u16
  T29 = typedef "TaskbarProgressAPI.lvlib/Progress State.ctl" = i32
  T30 = cluster{"t":dbl[], "Capacitance transient":dbl[]}
  T31 = cluster{"Clipboard":bool, "dat":bool, "iso":bool, "Origin":bool, "Excel":bool}
  T32 = cluster{"T_s 50%":dbl[unit], "T_s 1-1/e":dbl[unit], "T_s 90%":dbl[unit], "T_s 95%":dbl[unit], "T_s 99%":dbl[unit]}
  T33 = enum16{"Canceled", "Clipboard", "Dat", "Iso", "Origin", "Excel"}
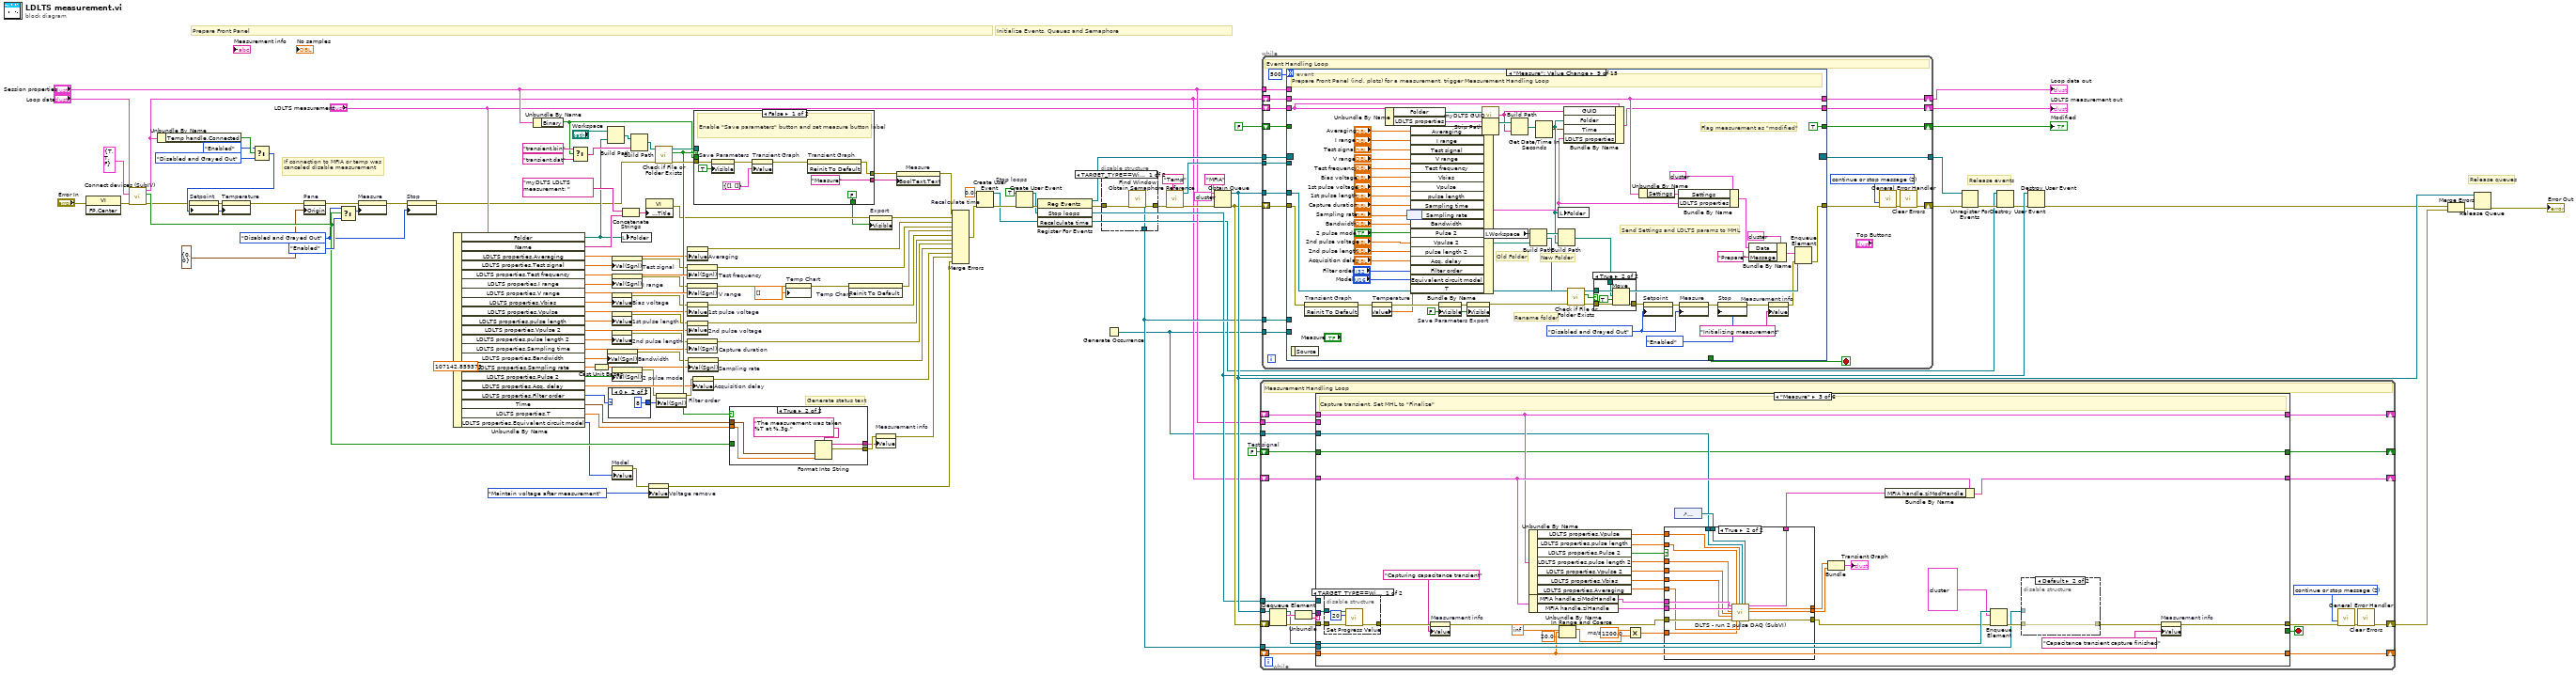
[diagram p0: block diagram]
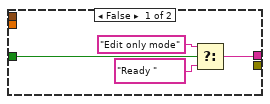
[diagram p4: hidden frame]
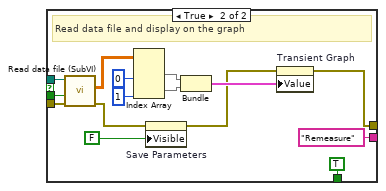
[diagram p5: hidden frame]
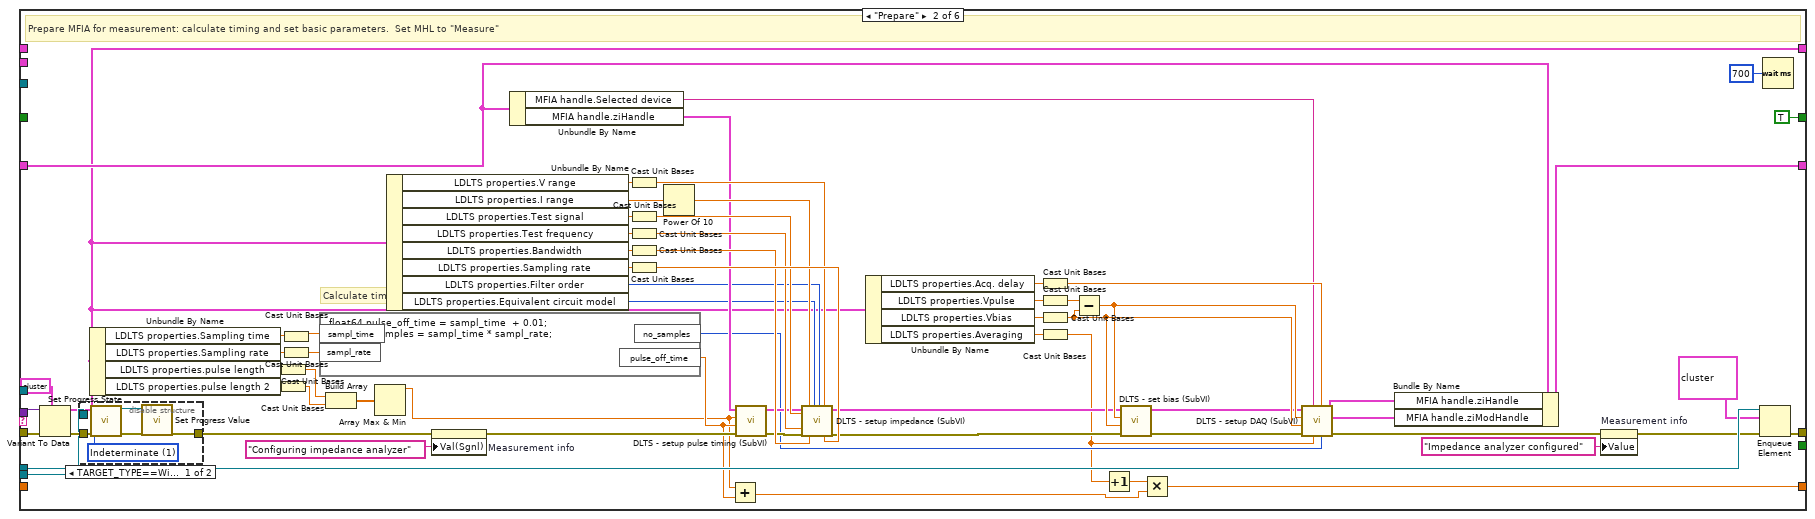
[diagram p7: hidden frame]
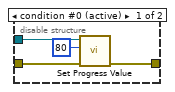
[diagram p9: hidden frame]
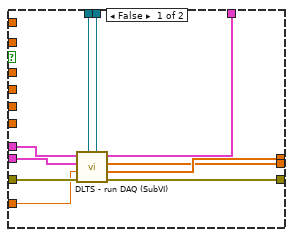
[diagram p11: hidden frame]
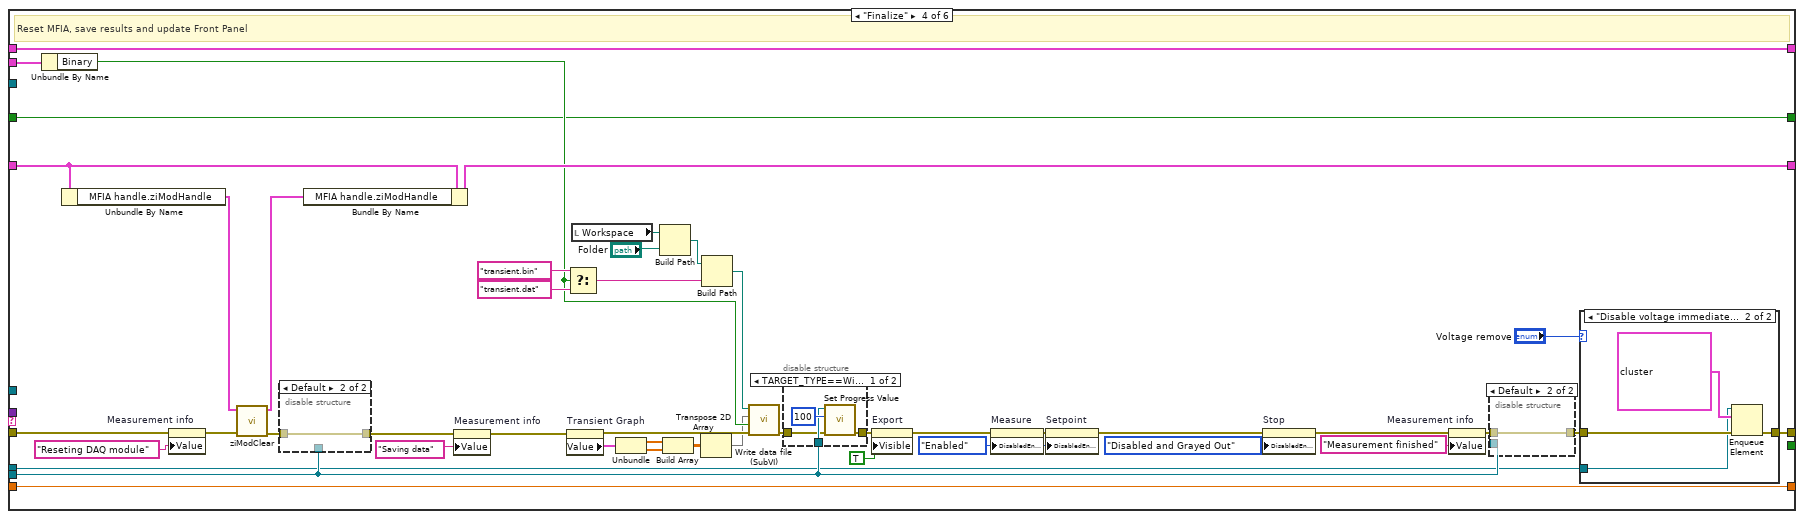
[diagram p12: hidden frame]
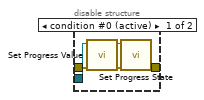
[diagram p13: hidden frame]
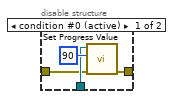
[diagram p15: hidden frame]
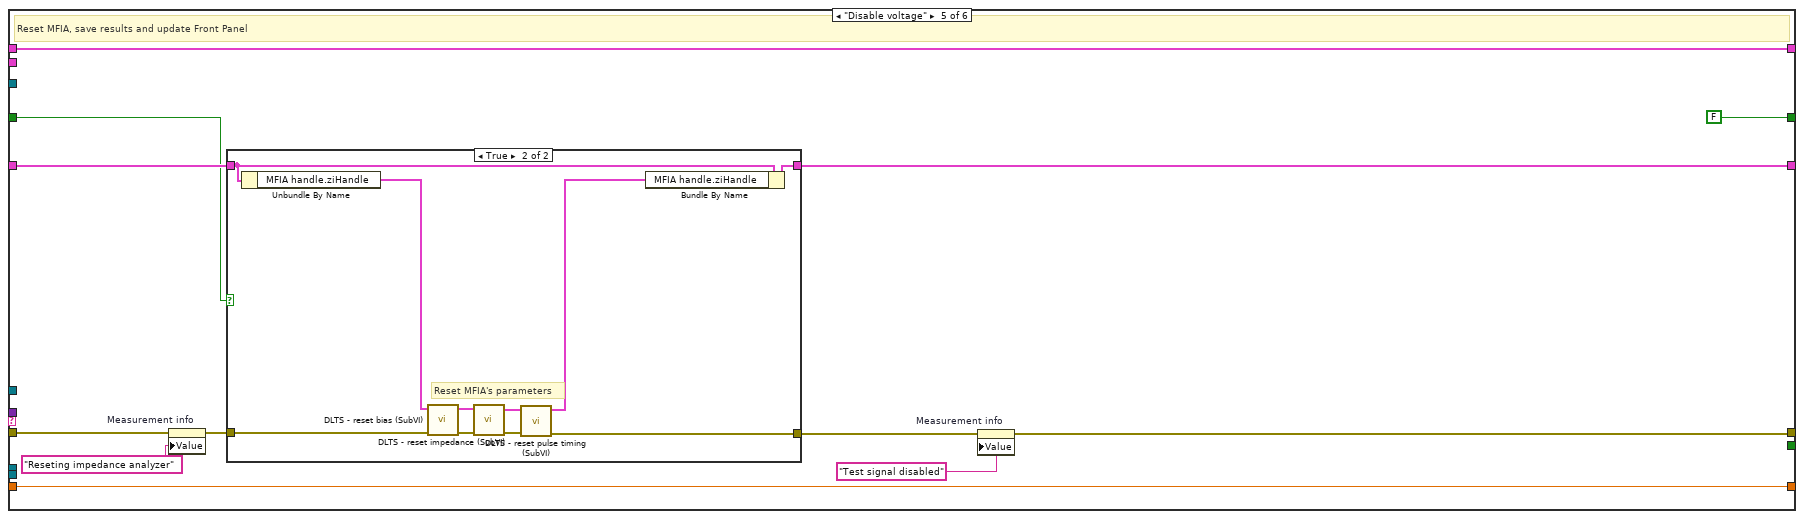
[diagram p17: hidden frame]
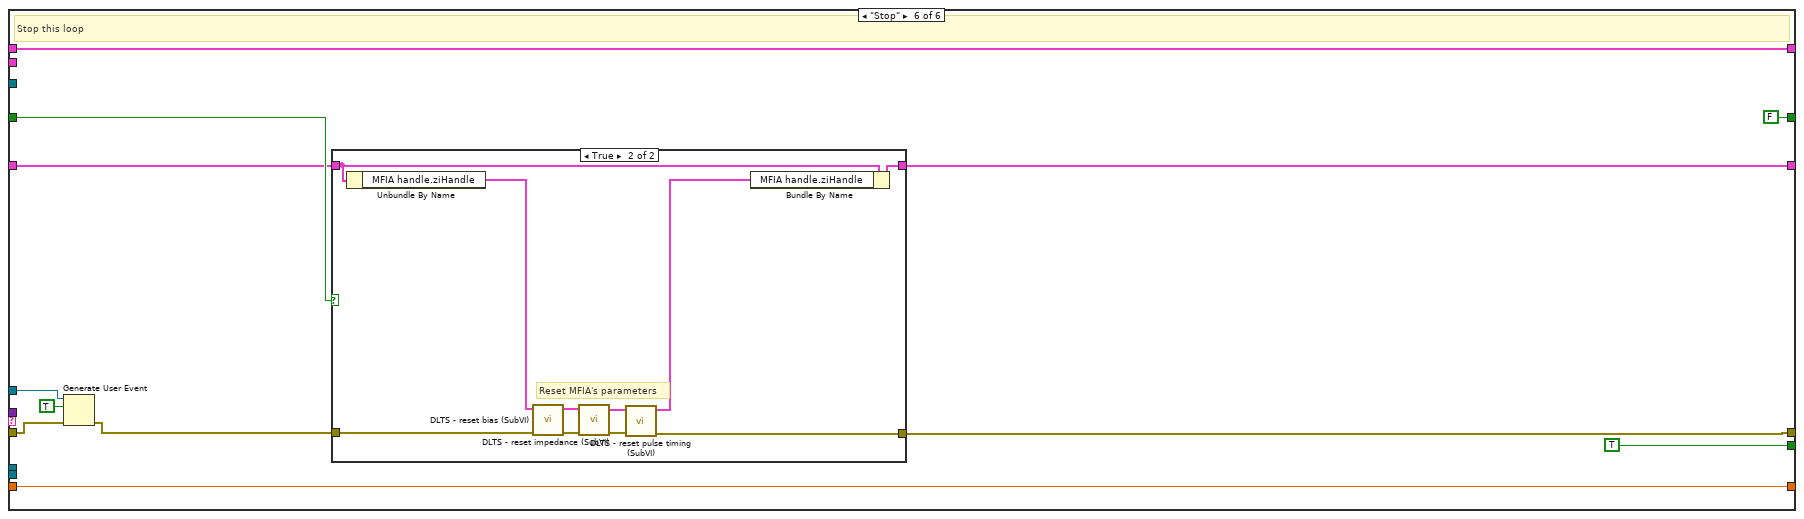
[diagram p19: hidden frame]
diagram:
  w10 = FALSE  # Test signal
  w42 = 0.0  # Recalculate time
  (unwired) dbl[unit] 107142.859375 ("Value (Signaling)")
  w104 = TRUE  # Stop loops
  w14 = T26."Disabled and Grayed Out" ("f")
  # "Release queues"
  # "Release events"
  # "Initialize Events, Queues and Semaphore"
  # "Generate status text"
  # "Prepare Front Panel"
  # "If connection to MFIA or temp was canceled disable measurement"
  n1 = invoke class="VI" method="FP.Center"(error in="Error In") -> (error out=w58:errorcluster)  [unwired: 2 in, 2 out]
  n2 = call "Connect devices (SubIV).vi"("Error In"=w58, "Devices"=T24 {"MFIA"=TRUE, "Temperature controller"=TRUE, "Source meter"=FALSE}, "Loop data in"="Loop data") -> ("Error Out"=w57:errorcluster, "Canceled"=w92:bool, "Loop data out"=w21:T6)  [unwired: 6 in]
  n3 = Unbundle By Name(w21) -> ("Temp handle.Connected"=w118:bool)
  n4 = Select(t=T26."Enabled" ("f"), s=w118, f=T26."Disabled and Grayed Out" ("Disabled")) -> (s? t:f=w76:T26)
  n5 = property on="Setpoint" class="DigNum (strict)"(error in=w57, "DisabledEnum"=w76) -> (error out=w119:errorcluster)  [unwired: 1 in, 1 out]
  n6 = property on="Temperature" class="DigNum (strict)"(error in=w119, "DisabledEnum"=w76) -> (error out=w20:errorcluster)  [unwired: 1 in, 1 out]
  n7 = property on="Pane" class="Pane"(error in=w20, "Origin"=T25 {"Horizontal"=0, "Vertical"=0}) -> (error out=w56:errorcluster)  [unwired: 1 in, 1 out]
  n8 = Select(t=w14, s=w92, f=T26."Enabled") -> (s? t:f=w115:T26)
  n9 = property on="Measure" class="Bool"(error in=w56, "DisabledEnum"=w115) -> (error out=w16:errorcluster)  [unwired: 1 in, 1 out]
  n10 = property on="Stop" class="Bool"(error in=w16, "DisabledEnum"=w14) -> (error out=w15:errorcluster)  [unwired: 1 in, 1 out]
  n11 = Unbundle By Name("LDLTS measurement") -> ("Folder"=w18:path, "Name"=w87:string, "LDLTS properties.Averaging"=w75:dbl, "LDLTS properties.Test signal"=w103:dbl[unit], "LDLTS properties.Test frequency"=w102:dbl[unit], "LDLTS properties.I range"=w101:dbl, "LDLTS properties.V range"=w100:dbl[unit], "LDLTS properties.Vbias"=w72:dbl[unit], "LDLTS properties.Vpulse"=w70:dbl[unit], "LDLTS properties.pulse length"=w69:dbl[unit], "LDLTS properties.Vpulse 2"=w32:dbl[unit], "LDLTS properties.pulse length 2"=w31:dbl[unit], "LDLTS properties.Sampling time"=w33:dbl[unit], "LDLTS properties.Bandwidth"=w55:dbl[unit], "LDLTS properties.Sampling rate"=w52:dbl[unit], "LDLTS properties.Pulse 2"=w34:bool, "LDLTS properties.Acq. delay"=w45:dbl[unit], "LDLTS properties.Filter order"=w13:i32, "Time"=w66:timestamp, "LDLTS properties.T"=w23:dbl[unit], "LDLTS properties.Equivalent circuit model"=w11:u16)
  n12 = Unbundle By Name("Session properties") -> ("Binary"=w50:bool)
  n13 = Select(t="transient.bin", s=w50, f="transient.dat") -> (s? t:f=w98:string)
  n14 = Cast Unit Bases(0:w52) -> (2:w51:dbl)  [unwired: 1 in]
  n15 = Build Path(base path="Workspace", name or relative path=w18) -> (appended path=w110:path)
  n16 = property on="Bandwidth" class="DigNum (strict)"("Val(Sgnl)"=w55) -> (error out=w53:errorcluster)  [unwired: 2 in, 1 out]
  n17 = case shown="0" w13 {
    selector: w13 -> [w121 _]
    tunnel: [w121 8 ("Filter order")] -> w12
    frame Default {
    }
    frame 0 {
    }
  }
  n18 = property on="Test signal" class="DigNum (strict)"("Val(Sgnl)"=w103) -> (error out=w73:errorcluster)  [unwired: 2 in, 1 out]
  n19 = property on="I range" class="Ring (strict)"("Val(Sgnl)"=w101) -> (error out=w74:errorcluster)  [unwired: 2 in, 1 out]
  n20 = property on="Bias voltage" class="DigNum (strict)"("Value"=w72) -> (error out=w71:errorcluster)  [unwired: 2 in, 1 out]
  n21 = property on="1st pulse length" class="DigNum (strict)"("Value"=w69) -> (error out=w30:errorcluster)  [unwired: 2 in, 1 out]
  n22 = property on="2nd pulse length" class="DigNum (strict)"("Value"=w31) -> (error out=w29:errorcluster)  [unwired: 2 in, 1 out]
  n23 = property on="2 pulse mode" class="Bool (strict)"("Val(Sgnl)"=w34) -> (error out=w8:errorcluster)  [unwired: 2 in, 1 out]
  n24 = property on="Model" class="Ring (strict)"("Value"=w11) -> (error out=w6:errorcluster)  [unwired: 2 in, 1 out]
  n25 = local write "Folder"(w18) -> ()
  n26 = Concatenate Strings("myDLTS LDLTS measurement: " ("string"), w87) -> (w88:string)
  n27 = Build Path(base path=w110, name or relative path=w98) -> (appended path=w109:path)
  n28 = property class="VI"("Front Panel.Title"=w88) -> (error out=w46:errorcluster)  [unwired: 2 in, 1 out]
  n29 = property on="Voltage remove" class="Enum (strict)"(error in=w6, "Value"=T1."Maintain voltage after measurement" ("Voltage remove")) -> (error out=w5:errorcluster)  [unwired: 1 in, 1 out]
  n30 = call <vilib>:"Check if File or Folder Exists.vi"("error in (no error)"=w15, "path"=w109) -> ("error out"=w107:errorcluster, "file or folder exists?"=w95:bool, "dup path"=w108:path)  [unwired: 7 in]
  n31 = property on="Filter order" class="DigNum (strict)"(error in=w8, "Val(Sgnl)"=w12) -> (error out=w7:errorcluster)  [unwired: 1 in, 1 out]
  n32 = property on="Averaging" class="DigNum (strict)"("Value"=w75) -> (error out=w68:errorcluster)  [unwired: 2 in, 1 out]
  n33 = property on="Test frequency" class="DigNum (strict)"(error in=w73, "Val(Sgnl)"=w102) -> (error out=w67:errorcluster)  [unwired: 1 in, 1 out]
  n34 = property on="V range" class="Ring (strict)"(error in=w74, "Val(Sgnl)"=w100) -> (error out=w4:errorcluster)  [unwired: 1 in, 1 out]
  n35 = property on="1st pulse voltage" class="DigNum (strict)"(error in=w71, "Value"=w70) -> (error out=w1:errorcluster)  [unwired: 1 in, 1 out]
  n36 = property on="2nd pulse voltage" class="DigNum (strict)"(error in=w30, "Value"=w32) -> (error out=w28:errorcluster)  [unwired: 1 in, 1 out]
  n37 = property on="Capture duration" class="DigNum (strict)"(error in=w29, "Val(Sgnl)"=w33) -> (error out=w27:errorcluster)  [unwired: 1 in, 1 out]
  n38 = property on="Sampling rate" class="Ring (strict)"(error in=w53, "Val(Sgnl)"=w51) -> (error out=w26:errorcluster)  [unwired: 1 in, 1 out]
  n39 = property on="Acquisition delay" class="DigNum (strict)"(error in=w7, "Value"=w45) -> (error out=w24:errorcluster)  [unwired: 1 in, 1 out]
  n40 = case shown="False" w95 {
    tunnel: w50 -> [_ w145]
    tunnel: w108 -> [_ w144]
    tunnel: w107 -> [w129 w143]
    tunnel: [w123 w132] -> w83
    tunnel: ["Measure" ("Boolean Text.Text") "Remeasure" ("Boolean Text.Text")] -> w81
    tunnel: [FALSE ("Visible") TRUE ("Visible")] -> w44
    frame False {
      # "Enable \"Save parameters\" button and set measure button label"
      n41 = property on="Save Parameters" class="Bool (strict)"(error in=w129, "Visible"=TRUE) -> (error out=w126:errorcluster)  [unwired: 1 in, 1 out]
      n42 = property on="Transient Graph" class="XYGraph (strict)"(error in=w126, "Value"=cluster{"t":dbl[], "Samples":dbl[]} {"t"=[], "Samples"=[]} ("Transient Graph")) -> (error out=w124:errorcluster)  [unwired: 1 in, 1 out]
      n43 = invoke on="Transient Graph" class="XYGraph (strict)" method="Reinit To Default"(error in=w124) -> (error out=w123:errorcluster)  [unwired: 2 in, 2 out]
    }
    frame True {
      # "Read data file and display on the graph"
      n44 = call "Read data file (SubVI).vi"("error in"=w143, "Binary"=w145, "file path in"=w144) -> ("error out"=w141:errorcluster, "2D data"=w136:dbl[][])  [unwired: 5 in, 2 out]
      n45 = Index Array(array=w136, index (col) #1=0 ("disabled index (col)"), index (col) #2=1 ("index (col)")) -> (element #1=w135:dbl[], element #2=w134:dbl[])  [unwired: 2 in]
      n46 = property on="Save Parameters" class="Bool (strict)"(error in=w141, "Visible"=FALSE) -> (error out=w131:errorcluster)  [unwired: 1 in, 1 out]
      n47 = Bundle("2D data"=w135, "2D data"=w134) -> (w133:cluster{"2D data":dbl[], "2D data":dbl[]})  [unwired: 1 in]
      n48 = property on="Transient Graph" class="XYGraph (strict)"(error in=w131, "Value"=w133) -> (error out=w132:errorcluster)  [unwired: 1 in, 1 out]
    }
  }
  n49 = case shown="True" w95 {
    tunnel: w66 -> [_ w154]
    tunnel: [_ w153] -> w94
    tunnel: [w148 w152] -> w93
    tunnel: w92 -> [w149 _]
    tunnel: w23 -> [_ w151]
    frame False {
      n50 = Select(t="Edit only mode", s=w149, f="Ready ") -> (s? t:f=w148:string)
    }
    frame True {
      n51 = Format Into String(format string="The measurement was taken %T at %.3g.", w154, w151) -> (resulting string=w152:string, error out=w153:errorcluster)  [unwired: 2 in]
    }
  }
  n52 = property on="Temp Chart" class="WFChart (strict)"(error in=w4, "History Data"=dbl[] []) -> (error out=w3:errorcluster)  [unwired: 1 in, 1 out]
  n53 = invoke on="Temp Chart" class="WFChart (strict)" method="Reinit To Default"(error in=w3) -> (error out=w54:errorcluster)  [unwired: 2 in, 2 out]
  n54 = property on="Export" class="Bool"(error in=w46, "Visible"=w44) -> (error out=w47:errorcluster)  [unwired: 1 in, 1 out]
  n55 = property on="Measurement info" class="Str"(error in=w94, "Value"=w93) -> (error out=w25:errorcluster)  [unwired: 1 in, 1 out]
  n56 = property on="Measure" class="Bool"(error in=w83, "BoolText.Text"=w81) -> (error out=w82:errorcluster)  [unwired: 1 in, 1 out]
  n57 = Merge Errors(w82, w47, w68, w67, w54, w1, w28, w27, w26, w24, w25, w5) -> (w40:errorcluster)
  n58 = Create User Event(user event datatype=w42, error in=w40) -> (user event=w37:refnum<user-event>, error out=w41:errorcluster)
  n59 = Create User Event(user event datatype=w104, error in=w41) -> (user event=w49:refnum<user-event>, error out=w105:errorcluster)
  n60 = register-events(error in=w105, w49, w37) -> (reference out=w106:refnum<event-registration>, error out=w61:errorcluster)  [unwired: 1 in]
  n61 = disable-structure shown="TARGET_TYPE==Windows" {
    disable-tunnel: w61 -> [w157 w158]
    disable-tunnel: [w156 _] -> w60
    disable-tunnel: [w155 w158] -> w22
    frame condition #0 (active) {
      n62 = call <vilib>:"Find Window.vi"("error in (no error)"=w157) -> ("error out"=w155:errorcluster, "Window Handle"=w156:refnum<k24>)  [unwired: 9 in]
    }
    frame condition #1 {
    }
  }
  n63 = Generate Occurrence() -> (w17:refnum<k4>)
  n64 = call <vilib>:"Obtain Semaphore Reference.vi"("error in (no error)"=w22, "name (unnamed)"="Temp") -> ("error out"=w65:errorcluster, "semaphore"=w63:T27)  [unwired: 3 in, 1 out]
  n65 = Obtain Queue(name (unnamed)="MFIA", element data type=cluster{"Data":variant, "Message":string} {"Data"=variant, "Message"=""}, error in (no error)=w65) -> (queue out=w89:refnum<queue>, error out=w62:errorcluster)  [unwired: 2 in, 1 out]
  n66 = while "Measurement Handling Loop" {
    tunnel: w89 -> [w174]
    shift-right: [w166] -> w77
    shift-left: w62 -> [w182]
    tunnel: w49 -> [w177]
    shift-right: [w173] -> _
    shift-left: w21 -> [w175]
    tunnel: w60 -> [w171]
    tunnel: "Session properties" -> [w167]
    shift-right: [w165] -> _
    shift-left: _ -> [w164]
    tunnel: w17 -> [w163]
    shift-right: [w162] -> _
    shift-left: _ -> [w161]
    shift-right: [w159] -> _
    shift-left: w10 -> [w160]
    stop <- w176 stop-if-true
    w168 = T28 2 items=["no dialog", "OK message", "continue or stop message", "OK message + warnings", "continue/stop + warnings"] ("type of dialog (OK msg:1)")
    # "Measurement Handling Loop"
    n67 = Dequeue Element(queue=w174, error in (no error)=w182) -> (queue out=w172:refnum<queue>, element=w181:cluster{"Data":variant, "Message":string}, error out=w178:errorcluster)  [unwired: 1 in, 1 out]
    n68 = Unbundle(w181) -> ("Data"=w179:variant, "Message"=w180:string)
    n69 = case shown="\"Measure\"" w180 {
      tunnel: w179 -> [_ w253 _ _ _ _]
      tunnel: w178 -> [w187 w254 w287 w370 w409 w436]
      tunnel: w177 -> [_ _ _ _ _ w435]
      tunnel: [w187 w208 w295 w336 w405 w427] -> w169
      tunnel: [_ _ _ _ _ TRUE] -> w176
      tunnel: w175 -> [w186 w246 w298 w379 w412 w429]
      tunnel: w172 -> [_ w249 w296 w335 _ _]
      tunnel: [w186 w245 w297 w378 w411 w426] -> w173
      tunnel: w171 -> [_ w243 w286 w364 _ _]
      tunnel: w167 -> [_ _ _ w357 _ _]
      tunnel: [w185 w197 w284 w347 w407 w432] -> w165
      tunnel: w164 -> [w185 _ w284 w347 w407 w432]
      tunnel: w163 -> [_ _ w272 _ _ _]
      tunnel: [w184 w194 w280 w340 w406 w431] -> w162
      tunnel: w161 -> [w184 _ w280 w340 w406 w431]
      tunnel: w160 -> [w183 _ w264 w339 w401 w430]
      tunnel: [w183 TRUE ("Test signal") w264 w339 FALSE ("Test signal") FALSE ("Test signal")] -> w159
      frame "", Default {
      }
      frame "Prepare" {
        # "Calculate timing"
        # "Prepare MFIA for measurement: calculate timing and set basic parameters.  Set MHL to \"Measure\""
        n70 = Variant To Data(error in=w254, type=cluster{"Settings":T12, "LDLTS properties":T3} {"Settings"={"MFIA"={"Address"="", "Use compensation"=TRUE, "Shut down gracefully"=FALSE}, "Temp ctrl"={"Gain (P)"=0.0, "Reset (I)"=0.0, "Rate (D)"=0.0, "Stabilization rate"=0.0, "Stabilization delta"=0.0, "Type"=enum."Lake Shore 325", "Custom temp ctrl"={"VISA resource name"=""}, "Lakeshore 325"={"VISA name"="", "Loop"=0, "Heater Range"=1, "Heater Resistance"=0, "Sample sensor"=0, "Fast sensor"=0, "Slow sensor"=0}, "Lakeshore 331"={"VISA name"="", "Loop"=1, "Heater Range"=0, "Sample sensor"=0, "Fast sensor"=0, "Slow sensor"=0}, "Lakeshore 332"={"VISA name"="", "Loop"=1, "Heater Range"=0, "Sample sensor"=0, "Fast sensor"=0, "Slow sensor"=0}, "Lakeshore 335"={"VISA name"="", "Loop"=1, "Sample sensor"=0, "Fast sensor"=0, "Slow sensor"=0, "Heater Range"=0, "Output mode"=enum."Off"}, "Lakeshore 336"={"VISA name"="", "Loop"=1, "Output mode"=enum."Off", "Max current"=1.0, "Heater resistance"=1, "Sample sensor"=1, "Slow sensor"=1, "Fast sensor"=1}}, "Source-meter"={"Type"=enum."Custom", "Custom source-meter"={"VISA resource name"=""}, "Keithley 2600"={"VISA name"="", "Ignore ID Query"=FALSE, "SMU"=enum."Channel A"}, "Keithley 2400 Series"={"VISA name"="", "Ignore ID Query"=FALSE}}, "Other"={"Enable OriginLab"=FALSE, "Reader mode"=FALSE, "Auto-save"=FALSE}, "Defaults"={"IV properties"={"T"=0.0, "Vstart"=-0.5, "Vstop"=0.5, "Vpoints"=10.0, "Settling"=0.01, "I limit"=0.1, "Log mapping"=FALSE, "Averaging"=0.0}, "CV properties"={"T"=0.0, "Vstart"=-0.5, "Vstop"=0.5, "Vpoints"=10.0, "Precision"=enum."Normal", "Test signal"=0.01, "Auto I range"=FALSE, "Test frequency"=100000.0, "I range"=-2.0, "V range"=10.0, "Log mapping"=FALSE, "Rel perm"=0.0, "Area"=0.0, "Equivalent circuit model"=0}, "DLTS properties"={"Tstart"=0.0, "Instant start"=FALSE, "Tstop"=0.0, "T rate"=0.0, "Test signal"=0.0, "Test frequency"=0.0, "Bandwidth"=0.0, "Averaging"=0.0, "Vbias"=0.0, "Vpulse"=0.0, "pulse length"=0.0, "Pulse 2"=FALSE, "Vpulse 2"=0.0, "pulse length 2"=0.0, "I range"=-2.0, "V range"=10.0, "Emission rate"=[], "Sampling rate"=0.0, "Acq. delay"=0.0, "Filter order"=0, "Equivalent circuit model"=0}, "LDLTS properties"={"T"=0.0, "Test signal"=0.0, "Test frequency"=0.0, "Bandwidth"=0.0, "Averaging"=0.0, "Vbias"=0.0, "Vpulse"=0.0, "pulse length"=0.0, "Pulse 2"=FALSE, "Vpulse 2"=0.0, "pulse length 2"=0.0, "I range"=-2.0, "V range"=10.0, "Sampling rate"=0.0, "Acq. delay"=0.0, "Sampling time"=0.0, "Filter order"=0, "Equivalent circuit model"=0}}}, "LDLTS properties"={"T"=0.0, "Test signal"=0.0, "Test frequency"=0.0, "Bandwidth"=0.0, "Averaging"=0.0, "Vbias"=0.0, "Vpulse"=0.0, "pulse length"=0.0, "Pulse 2"=FALSE, "Vpulse 2"=0.0, "pulse length 2"=0.0, "I range"=-2.0, "V range"=10.0, "Sampling rate"=0.0, "Acq. delay"=0.0, "Sampling time"=0.0, "Filter order"=0, "Equivalent circuit model"=0}}, Variant=w253) -> (data=w194:cluster{"Settings":T12, "LDLTS properties":T3}, error out=w244:errorcluster)
        n71 = disable-structure shown="TARGET_TYPE==Windows" {
          disable-tunnel: w244 -> [w260 w261]
          disable-tunnel: w243 -> [w259 _]
          disable-tunnel: [w255 w261] -> w206
          frame condition #0 (active) {
            w258 = T29 1 items=["NoProgress"=0, "Indeterminate"=1, "Normal"=2, "Error"=4, "Paused"=8] ("State (No Progress)")
            n72 = call <vilib>:"Set Progress State.vi"("error in (no error)"=w260, "State (No Progress)"=w258, "Window Handle"=w259) -> ("error out"=w257:errorcluster, "dup Window Handle"=w256:refnum<k24>)  [unwired: 7 in]
            n73 = call <vilib>:"Set Progress Value.vi"("error in (no error)"=w257, "Window Handle"=w256) -> ("error out"=w255:errorcluster)  [unwired: 8 in, 1 out]
          }
          frame condition #1 {
          }
        }
        n74 = Unbundle By Name(w194) -> ("LDLTS properties.Sampling time"=w238:dbl[unit], "LDLTS properties.Sampling rate"=w239:dbl[unit], "LDLTS properties.pulse length"=w240:dbl[unit], "LDLTS properties.pulse length 2"=w192:dbl[unit])
        n75 = Cast Unit Bases(0:w240) -> (2:w190:dbl)  [unwired: 1 in]
        n76 = Cast Unit Bases(0:w192) -> (2:w191:dbl)  [unwired: 1 in]
        n77 = Cast Unit Bases(0:w238) -> (2:w241:dbl)  [unwired: 1 in]
        n78 = Cast Unit Bases(0:w239) -> (2:w242:dbl)  [unwired: 1 in]
        n79 = formula code="float64 pulse_off_time = sampl_time  + 0.01;\nint32 no_samples = sampl_time * sampl_rate;"("sampl_time"=w241, "sampl_rate"=w242) -> ("pulse_off_time"=w202:dbl, "no_samples"=w201:i32)
        n80 = Build Array(w190, w191) -> (w189:dbl[])
        n81 = Array Max & Min(array=w189) -> (max value=w188:dbl)  [unwired: 3 out]
        n82 = Unbundle By Name(w194) -> ("LDLTS properties.V range"=w225:dbl[unit], "LDLTS properties.I range"=w230:dbl, "LDLTS properties.Test signal"=w226:dbl[unit], "LDLTS properties.Test frequency"=w227:dbl[unit], "LDLTS properties.Bandwidth"=w228:dbl[unit], "LDLTS properties.Sampling rate"=w229:dbl[unit], "LDLTS properties.Filter order"=w196:i32, "LDLTS properties.Equivalent circuit model"=w195:u16)
        n83 = property on="Measurement info" class="Str"(error in=w206, "Val(Sgnl)"="Configuring impedance analyzer" ("Value (Signaling)")) -> (error out=w237:errorcluster)  [unwired: 1 in, 1 out]
        n84 = Unbundle By Name(w246) -> ("MFIA handle.Selected device"=w203:string, "MFIA handle.ziHandle"=w222:T21)
        n85 = Cast Unit Bases(0:w225) -> (2:w231:dbl)  [unwired: 1 in]
        n86 = Cast Unit Bases(0:w226) -> (2:w233:dbl)  [unwired: 1 in]
        n87 = Cast Unit Bases(0:w227) -> (2:w234:dbl)  [unwired: 1 in]
        n88 = Cast Unit Bases(0:w228) -> (2:w235:dbl)  [unwired: 1 in]
        n89 = Cast Unit Bases(0:w229) -> (2:w236:dbl)  [unwired: 1 in]
        n90 = Power Of 10(x=w230) -> (10^x=w232:dbl)
        n91 = Add(x=w188, y=w202) -> (x+y=w199:dbl)
        n92 = call "DLTS - setup pulse timing (SubVI).vi"("error in (no error)"=w237, "TUpulse off time"=w202, "TUpulse on time"=w188, "Handle Out in"=w222) -> ("error out"=w224:errorcluster, "Handle Out out"=w223:T21)  [unwired: 6 in]
        n93 = call "DLTS - setup impedance (SubVI).vi"("Handle Out in"=w223, "IMPS test signal"=w233, "IMPS test freq"=w234, "error in (no error)"=w224, "IMPS current range"=w232, "IMPS  bandwidth"=w235, "Equivalent circuit model"=w195, "Filter order"=w196, "IMPS output range"=w231, "IMPS demod sampling rate"=w236) -> ("Handle Out out"=w212:T21, "error out"=w213:errorcluster)  [unwired: 8 in]
        n94 = Unbundle By Name(w194) -> ("LDLTS properties.Acq. delay"=w214:dbl[unit], "LDLTS properties.Vpulse"=w215:dbl[unit], "LDLTS properties.Vbias"=w216:dbl[unit], "LDLTS properties.Averaging"=w217:dbl)
        n95 = Cast Unit Bases(0:w214) -> (2:w219:dbl)  [unwired: 1 in]
        n96 = Cast Unit Bases(0:w215) -> (2:w218:dbl)  [unwired: 1 in]
        n97 = Cast Unit Bases(0:w216) -> (2:w221:dbl)  [unwired: 1 in]
        n98 = Cast Unit Bases(0:w217) -> (2:w198:dbl)  [unwired: 1 in]
        n99 = Subtract(x=w218, y=w221) -> (x-y=w220:dbl)
        n100 = Increment(x=w198) -> (x+1=w200:dbl)
        n101 = call "DLTS - set bias (SubVI).vi"("error in (no error)"=w213, "AUX offset"=w221, "AUX scale"=w220, "ziHandle"=w212) -> ("error out"=w204:errorcluster, "Handle Out"=w205:T21)  [unwired: 6 in]
        n102 = Multiply(x=w200, y=w199) -> (x*y=w197:dbl)
        n103 = call "DLTS - setup DAQ (SubVI).vi"("No. samples"=w201, "post trigger delay"=w219, "No. repetitions (avg)"=w198, "Selected device"=w203, "error in (no error)"=w204, "AUX offset"=w221, "AUX scale"=w220, "Handle in"=w205) -> ("error out"=w209:errorcluster, "ModHandle Out"=w210:T22, "Handle Out"=w211:T21)  [unwired: 1 in]
        n104 = Bundle By Name(cluster=w246, "MFIA handle.ziHandle"=w211, "MFIA handle.ziModHandle"=w210) -> (w245:T6)
        n105 = property on="Measurement info" class="Str"(error in=w209, "Value"="Impedance analyzer configured" ("Measurement info")) -> (error out=w248:errorcluster)  [unwired: 1 in, 1 out]
        n106 = Enqueue Element(queue=w249, element=cluster{"Data":variant, "Message":string} {"Data"=variant, "Message"="Measure"}, error in (no error)=w248) -> (error out=w208:errorcluster)  [unwired: 1 in, 2 out]
        n107 = Wait (ms)(milliseconds to wait=u32 700) -> ()  [unwired: 1 out]
      }
      frame "Measure" {
        w285 = 1200.0  # ms/s
        # "Capture transient. Set MHL to \"Finalize\""
        n108 = disable-structure shown="TARGET_TYPE==Windows" {
          disable-tunnel: [w306 w308] -> w289
          disable-tunnel: w287 -> [w305 w308]
          disable-tunnel: w286 -> [w304 _]
          frame condition #0 (active) {
            n109 = call <vilib>:"Set Progress Value.vi"("error in (no error)"=w305, "current (0)"=u64 20, "Window Handle"=w304) -> ("error out"=w306:errorcluster)  [unwired: 7 in, 1 out]
          }
          frame condition #1 {
          }
        }
        n110 = property on="Measurement info" class="Str"(error in=w289, "Value"="Capturing capacitance transient" ("Measurement info")) -> (error out=w278:errorcluster)  [unwired: 1 in, 1 out]
        n111 = Unbundle By Name(w280) -> ("LDLTS properties.Vpulse"=w262:dbl[unit], "LDLTS properties.pulse length"=w271:dbl[unit], "LDLTS properties.Pulse 2"=w270:bool, "LDLTS properties.pulse length 2"=w269:dbl[unit], "LDLTS properties.Vpulse 2"=w268:dbl[unit], "LDLTS properties.Vbias"=w267:dbl[unit], "LDLTS properties.Averaging"=w263:dbl)
        n112 = Unbundle By Name(w298) -> ("MFIA handle.ziModHandle"=w266:T22, "MFIA handle.ziHandle"=w265:T21)
        n113 = In Range and Coerce(upper limit=inf, x=w284, lower limit=20.0) -> (coerced(x)=w283:dbl)  [unwired: 1 out]
        n114 = Multiply(x=w285, y=w283) -> (x*y=w277:dbl)
        n115 = control-ref of="Measurement info"() -> (w279:refnum<vi>)
        n116 = case shown="True" w270 {
          tunnel: w278 -> [w318 w334]
          tunnel: w266 -> [w317 w332]
          tunnel: w265 -> [w316 w331]
          tunnel: [w315 w326] -> w273
          tunnel: [w314 w333] -> w276
          tunnel: [w313 w327] -> w274
          tunnel: [w312 w328] -> w275
          tunnel: w269 -> [_ w321]
          tunnel: w271 -> [_ w322]
          tunnel: w268 -> [_ w320]
          tunnel: w267 -> [_ w319]
          tunnel: w279 -> [w311 w325]
          tunnel: w277 -> [w309 w329]
          tunnel: w272 -> [w310 w324]
          tunnel: w263 -> [_ w330]
          tunnel: w262 -> [_ w323]
          frame False {
            n117 = call "DLTS - run DAQ (SubVI).vi"("Status String Reference"=w311, "Abort Occurrence"=w310, "error in (no error)"=w318, "Timeout 5000ms"=w309, "Handle in"=w316, "ModHandle in"=w317) -> ("error out"=w314:errorcluster, "t"=w313:dbl[], "Samples"=w312:dbl[], "ModHandle Out  out"=w315:T22)  [unwired: 1 in, 1 out]
          }
          frame True {
            n118 = call "DLTS - run 2 pulse DAQ (SubVI).vi"("ziModHandle"=w332, "ziHandle"=w331, "pulse length 2"=w321, "Vpulse 2"=w320, "Vbias"=w319, "error in (no error)"=w334, "pulse length"=w322, "Timeout"=w329, "Vpulse"=w323, "Averaging"=w330, "occurrence"=w324, "Status string"=w325) -> ("ModHandle Out"=w326:T22, "t"=w327:dbl[], "Capacitance transient"=w328:dbl[], "error out"=w333:errorcluster)  [unwired: 4 in]
          }
        }
        n119 = Bundle("t"=w274, "Capacitance transient"=w275) -> (→"Transient Graph":T30)  [unwired: 1 in]
        n120 = Bundle By Name(cluster=w298, "MFIA handle.ziModHandle"=w273) -> (w297:T6)
        n121 = Enqueue Element(queue=w296, element=cluster{"Data":variant, "Message":string} {"Data"=variant, "Message"="Finalize"}, error in (no error)=w276) -> (error out=w293:errorcluster)  [unwired: 1 in, 2 out]
        n122 = disable-structure shown="Default" {
          disable-tunnel: w293 -> [w302 w303]
          disable-tunnel: [w300 w303] -> w291
          disable-tunnel: w286 -> [w299 _]
          frame condition #0 (active) {
            n123 = call <vilib>:"Set Progress Value.vi"("error in (no error)"=w302, "current (0)"=u64 80, "Window Handle"=w299) -> ("error out"=w300:errorcluster)  [unwired: 7 in, 1 out]
          }
          frame condition #1 {
          }
        }
        n124 = property on="Measurement info" class="Str"(error in=w291, "Value"="Capacitance transient capture finished" ("Measurement info")) -> (error out=w295:errorcluster)  [unwired: 1 in, 1 out]
      }
      frame "Finalize" {
        w375 = T26."Enabled" ("Disabled")
        # "Reset MFIA, save results and update Front Panel"
        n125 = Unbundle By Name(w357) -> ("Binary"=w355:bool)
        n126 = Unbundle By Name(w379) -> ("MFIA handle.ziModHandle"=w342:T22)
        n127 = property on="Measurement info" class="Str"(error in=w370, "Value"="Reseting DAQ module" ("Measurement info")) -> (error out=w369:errorcluster)  [unwired: 1 in, 1 out]
        n128 = call <instrlib>:"ziModClear.vi"("Error In"=w369, "ziModHandle In"=w342) -> ("Error Out"=w343:errorcluster, "ModHandle Out"=w341:T22)  [unwired: 7 in]
        n129 = disable-structure shown="Default" {
          disable-tunnel: [w393 w395] -> w368
          disable-tunnel: w364 -> [w392 _]
          disable-tunnel: w343 -> [w391 w395]
          frame condition #0 (active) {
            n130 = call <vilib>:"Set Progress Value.vi"("error in (no error)"=w391, "current (0)"=u64 90, "Window Handle"=w392) -> ("error out"=w393:errorcluster)  [unwired: 7 in, 1 out]
          }
          frame condition #1 {
          }
        }
        n131 = Bundle By Name(cluster=w379, "MFIA handle.ziModHandle"=w341) -> (w378:T6)
        n132 = property on="Measurement info" class="Str"(error in=w368, "Value"="Saving data" ("Measurement info")) -> (error out=w367:errorcluster)  [unwired: 1 in, 1 out]
        n133 = property on="Transient Graph" class="XYGraph (strict)"(error in=w367) -> (error out=w354:errorcluster, "Value"=w352:cluster{"t":dbl[], "Samples":dbl[]})  [unwired: 1 in, 1 out]
        n134 = Select(t="transient.bin", s=w355, f="transient.dat") -> (s? t:f=w361:string)
        n135 = local read "Workspace"() -> (w359:path)
        n136 = Unbundle(w352) -> ("t"=w351:dbl[], "Samples"=w350:dbl[])
        n137 = Build Path(base path=w359, name or relative path="Folder") -> (appended path=w362:path)
        n138 = Build Array(w351, w350) -> (w353:dbl[][])
        n139 = Transpose 2D Array(2D array=w353) -> (transposed array=w349:dbl[][])
        n140 = Build Path(base path=w362, name or relative path=w361) -> (appended path=w358:path)
        n141 = call "Write data file (SubVI).vi"("error in"=w354, "Binary"=w355, "2D data"=w349, "file path in"=w358) -> ("error out"=w363:errorcluster)  [unwired: 6 in, 1 out]
        n142 = disable-structure shown="TARGET_TYPE==Windows" {
          disable-tunnel: [w388 w390] -> w365
          disable-tunnel: w364 -> [w387 _]
          disable-tunnel: w363 -> [w386 w390]
          frame condition #0 (active) {
            n143 = call <vilib>:"Set Progress Value.vi"("error in (no error)"=w386, "current (0)"=u64 100, "Window Handle"=w387) -> ("error out"=w388:errorcluster)  [unwired: 7 in, 1 out]
          }
          frame condition #1 {
          }
        }
        n144 = property on="Export" class="Bool"(error in=w365, "Visible"=TRUE) -> (error out=w366:errorcluster)  [unwired: 1 in, 1 out]
        n145 = property on="Measure" class="Bool"(error in=w366, "DisabledEnum"=w375) -> (error out=w374:errorcluster)  [unwired: 1 in, 1 out]
        n146 = property on="Setpoint" class="DigNum (strict)"(error in=w374, "DisabledEnum"=w375) -> (error out=w346:errorcluster)  [unwired: 1 in, 1 out]
        n147 = property on="Stop" class="Bool"(error in=w346, "DisabledEnum"=T26."Disabled and Grayed Out" ("Disabled")) -> (error out=w345:errorcluster)  [unwired: 1 in, 1 out]
        n148 = property on="Measurement info" class="Str"(error in=w345, "Value"="Measurement finished" ("Measurement info")) -> (error out=w377:errorcluster)  [unwired: 1 in, 1 out]
        n149 = disable-structure shown="Default" {
          disable-tunnel: w377 -> [w382 w385]
          disable-tunnel: w364 -> [w381 _]
          disable-tunnel: [w380 w385] -> w337
          frame condition #0 (active) {
            n150 = call <vilib>:"Set Progress Value.vi"("error in (no error)"=w382, "Window Handle"=w381) -> ("error out"=w383:errorcluster, "dup Window Handle"=w384:refnum<k24>)  [unwired: 8 in]
            n151 = call <vilib>:"Set Progress State.vi"("error in (no error)"=w383, "Window Handle"=w384) -> ("error out"=w380:errorcluster)  [unwired: 8 in, 1 out]
          }
          frame condition #1 {
          }
        }
        n152 = case shown="\"Disable voltage immediately after measurement\"" "Voltage remove" {
          tunnel: w337 -> [w396 w399]
          tunnel: [w396 w398] -> w336
          tunnel: w335 -> [_ w397]
          frame "Maintain voltage after measurement", Default {
          }
          frame "Disable voltage immediately after measurement" {
            n153 = Enqueue Element(queue=w397, element=cluster{"Data":variant, "Message":string} {"Data"=variant, "Message"="Disable voltage"}, error in (no error)=w399) -> (error out=w398:errorcluster)  [unwired: 1 in, 2 out]
          }
        }
      }
      frame "Disable voltage" {
        # "Reset MFIA, save results and update Front Panel"
        n154 = property on="Measurement info" class="Str"(error in=w409, "Value"="Reseting impedance analyzer" ("Measurement info")) -> (error out=w408:errorcluster)  [unwired: 1 in, 1 out]
        n155 = case shown="True" w401 {
          tunnel: w412 -> [w413 w418]
          tunnel: [w413 w417] -> w411
          tunnel: w408 -> [w414 w416]
          tunnel: [w414 w415] -> w404
          frame False {
          }
          frame True {
            # "Reset MFIA's parameters"
            n156 = Unbundle By Name(w418) -> ("MFIA handle.ziHandle"=w420:T21)
            n157 = call "DLTS - reset bias (SubVI).vi"("error in (no error)"=w416, "Handle in"=w420) -> ("error out"=w424:errorcluster, "Handle out"=w423:T21)  [unwired: 8 in]
            n158 = call "DLTS - reset impedance (SubVI).vi"("error in (no error)"=w424, "Handle in"=w423) -> ("error out"=w422:errorcluster, "Handle out"=w421:T21)  [unwired: 8 in]
            n159 = call "DLTS - reset pulse timing (SubVI).vi"("error in (no error)"=w422, "Handle in"=w421) -> ("error out"=w415:errorcluster, "Handle out"=w419:T21)  [unwired: 8 in]
            n160 = Bundle By Name(cluster=w418, "MFIA handle.ziHandle"=w419) -> (w417:T6)
          }
        }
        n161 = property on="Measurement info" class="Str"(error in=w404, "Value"="Test signal disabled" ("Measurement info")) -> (error out=w405:errorcluster)  [unwired: 1 in, 1 out]
      }
      frame "Stop" {
        # "Stop this loop"
        n162 = Generate User Event(user event=w435, event data cluster=TRUE ("event data"), error in=w436) -> (error out=w428:errorcluster)  [unwired: 1 in, 1 out]
        n163 = case shown="True" w430 {
          tunnel: w429 -> [w437 w442]
          tunnel: [w437 w441] -> w426
          tunnel: w428 -> [w438 w440]
          tunnel: [w438 w439] -> w427
          frame False {
          }
          frame True {
            # "Reset MFIA's parameters"
            n164 = Unbundle By Name(w442) -> ("MFIA handle.ziHandle"=w444:T21)
            n165 = call "DLTS - reset bias (SubVI).vi"("error in (no error)"=w440, "Handle in"=w444) -> ("error out"=w448:errorcluster, "Handle out"=w447:T21)  [unwired: 8 in]
            n166 = call "DLTS - reset impedance (SubVI).vi"("error in (no error)"=w448, "Handle in"=w447) -> ("error out"=w446:errorcluster, "Handle out"=w445:T21)  [unwired: 8 in]
            n167 = call "DLTS - reset pulse timing (SubVI).vi"("error in (no error)"=w446, "Handle in"=w445) -> ("error out"=w439:errorcluster, "Handle out"=w443:T21)  [unwired: 8 in]
            n168 = Bundle By Name(cluster=w442, "MFIA handle.ziHandle"=w443) -> (w441:T6)
          }
        }
      }
    }
    n169 = call <vilib>:"General Error Handler.vi"("type of dialog (OK msg:1)"=w168, "error in (no error)"=w169) -> ("error out"=w170:errorcluster)  [unwired: 9 in, 4 out]
    n170 = call <vilib>:"Clear Errors.vi"("error in (no error)"=w170) -> ("error out"=w166:errorcluster)  [unwired: 5 in, 1 out]
  }
  n171 = while "Event Handling Loop" {
    shift-right: [w463] -> w113
    shift-left: w21 -> [w466]
    shift-right: [w464] -> w35
    shift-left: "LDLTS measurement" -> [w465]
    shift-right: [w450] -> w91
    shift-left: w62 -> [w467]
    tunnel: w89 -> [w462]
    tunnel: w106 -> [w461]
    tunnel: [w460] -> w90
    shift-right: [w458] -> w84
    shift-left: FALSE -> [w459]
    tunnel: w63 -> [w457]
    tunnel: w60 -> [w456]
    tunnel: "Session properties" -> [w451]
    tunnel: w17 -> [w449]
    stop <- w468 stop-if-true
    w452 = T28 2 items=["no dialog", "OK message", "continue or stop message", "OK message + warnings", "continue/stop + warnings"] ("type of dialog (OK msg:1)")
    # "Event Handling Loop"
    n172 = event shown="[8] \"Measure\": Value Change" {
      selector: w461 -> [_ _ _ _ _ _ _ _ _ _ _ _ _ _ _]
      dyn-events: [_ _ _ _ _ _ _ _ _ _ _ _ _ _ _] -> w460
      timeout: 500 -> [_ _ _ _ _ _ _ _ _ _ _ _ _ _ _]
      tunnel: [_ TRUE _ _ _ _ _ _ _ _ _ _ _ _ _] -> w468
      tunnel: w467 -> [w475 w498 w509 w525 w535 w549 w559 w567 w577 w643 w648 w652 w685 w718 w753]
      tunnel: w466 -> [w471 w505 w513 w522 w538 w552 w561 w565 w631 w644 w649 w665 w689 w724 w751]
      tunnel: w465 -> [w476 w506 w514 w523 w541 w551 w562 w564 w618 w645 w650 w666 w688 w722 w756]
      tunnel: [w476 w506 w514 w523 w541 w551 w562 w564 w616 w645 w650 w666 w687 w721 w756] -> w464
      tunnel: [w471 w505 w513 w522 w538 w552 w561 w565 w631 w644 w649 w665 w689 w724 w751] -> w463
      tunnel: [w474 w504 w512 w524 w532 w547 w557 w566 w627 w643 w648 w653 w684 w717 w757] -> w453
      tunnel: w462 -> [_ w502 w510 _ _ _ _ _ w625 _ _ _ _ _ _]
      tunnel: w459 -> [w473 w503 w511 w521 w540 w550 w560 w563 _ w642 w647 w664 w682 w719 w758]
      tunnel: [w473 w503 w511 w521 w540 w550 w560 w563 TRUE w642 w647 w664 w686 w720 w758] -> w458
      tunnel: w457 -> [w472 _ _ _ w536 _ _ _ _ _ _ _ _ _ _]
      tunnel: w456 -> [_ _ _ _ _ _ _ _ _ _ _ _ _ _ _]
      tunnel: w451 -> [_ _ _ _ _ _ _ _ _ _ _ _ _ _ w755]
      tunnel: w449 -> [_ _ _ _ _ _ _ _ _ _ w646 _ _ _ _]
      event Timeout {
        # "Refresh temperature and setpoint reading on Front Panel"
        n173 = event-data() -> ()  [unwired: 1 in, 1 out]
        n174 = Unbundle By Name(w471) -> ("Temp handle"=w470:T8, "Temp handle.Connected"=w469:bool)
        n175 = case shown="True" w469 {
          tunnel: w475 -> [w477 w490]
          tunnel: [w477 w489] -> w474
          tunnel: w472 -> [_ w488]
          tunnel: w470 -> [_ w484]
          frame False {
          }
          frame True {
            n176 = call <vilib>:"Acquire Semaphore.vi"("error in (no error)"=w490, "semaphore"=w488) -> ("error out"=w483:errorcluster, "semaphore out"=w485:T27)  [unwired: 3 in, 1 out]
            n177 = call "Temp ctrl - Read temp and stp.vi"("Error In"=w483, "Temp handle"=w484) -> ("Error Out"=w479:errorcluster, "Sample temperature"=w482:dbl[unit], "Setpoint"=w478:dbl[unit])  [unwired: 2 in, 2 out]
            "Temperature" <- w482
            n178 = Cast Unit Bases(0:w482) -> (2:→"Temp Chart":dbl)  [unwired: 1 in]
            n179 = property on="Setpoint" class="DigNum (strict)"(error in=w479) -> (error out=w487:errorcluster, "Key Focus"=w480:bool)  [unwired: 1 in, 1 out]
            n180 = case shown="False" w480 {
              tunnel: w487 -> [w492 w494]
              tunnel: [w493 w494] -> w486
              tunnel: w478 -> [w491 _]
              frame False {
                # "Update setpoint if not currently edited"
                n181 = property on="Setpoint" class="DigNum (strict)"(error in=w492, "Value"=w491) -> (error out=w493:errorcluster)  [unwired: 1 in, 1 out]
              }
              frame True {
              }
            }
            n182 = call <vilib>:"Release Semaphore.vi"("error in (no error)"=w486, "semaphore"=w485) -> ("error out"=w489:errorcluster)  [unwired: 4 in, 1 out]
          }
        }
      }
      event Panel Close? {
        # "Check whether measurement and analysis are finished: if yes stop the loop, if no display dialog"
        n183 = event-data() -> ()  [unwired: 1 in, 1 out]
        n184 = Get Queue Status(queue=w502, error in (no error)=w498) -> (queue out=w501:refnum<queue>, error out=w500:errorcluster)  [unwired: 1 in, 6 out]
        n185 = Bundle By Name(cluster=cluster{"Data":variant, "Message":string} {"Data"=variant, "Message"=""}, "Message"="Stop") -> (w496:cluster{"Data":variant, "Message":string})
        n186 = Enqueue Element(queue=w501, element=w496, error in (no error)=w500) -> (error out=w504:errorcluster)  [unwired: 1 in, 2 out]
        n187 = event-data("Discard?"=TRUE) -> ()  [unwired: 1 in, 1 out]
      }
      event "Voltage remove": Value Change {
        # "Check whether measurement and analysis are finished: if yes stop the loop, if no display dialog"
        n188 = event-data() -> ("NewVal"=w508:T1)  [unwired: 1 in]
        n189 = case shown="\"Disable voltage immediately after measurement\"" w508 {
          tunnel: [w515 w519] -> w512
          tunnel: w510 -> [_ w518]
          tunnel: w509 -> [w515 w517]
          frame "Maintain voltage after measurement", Default {
          }
          frame "Disable voltage immediately after measurement" {
            n190 = Enqueue Element(queue=w518, element=cluster{"Data":variant, "Message":string} {"Data"=variant, "Message"="Disable voltage"}, error in (no error)=w517) -> (error out=w519:errorcluster)  [unwired: 1 in, 2 out]
          }
        }
      }
      event "Top Buttons.Help": Value Change {
        n191 = event-data() -> ("NewVal"=w520:bool)  [unwired: 1 in]
        n192 = case shown="True" w520 {
          tunnel: w525 -> [w526 w530]
          tunnel: [w526 w529] -> w524
          tunnel: w522 -> [_ w528]
          frame False {
          }
          frame True {
            n193 = Unbundle By Name(w528) -> ("Paths.Manual"=w527:path)
            n194 = call "OpenDoc Browser.vi"("error in (no error)"=w530, "File"=w527) -> ("error out"=w529:errorcluster)  [unwired: 9 in]
          }
        }
      }
      event "Setpoint": Value Change {
        # "Update temperature setpoint"
        n195 = event-data() -> ()  [unwired: 1 in, 1 out]
        n196 = call <vilib>:"Acquire Semaphore.vi"("error in (no error)"=w535, "semaphore"=w536) -> ("error out"=w534:errorcluster, "semaphore out"=w531:T27)  [unwired: 3 in, 1 out]
        n197 = Unbundle By Name(w538) -> ("Temp handle"=w537:T8)
        n198 = call "Temp ctrl - Setpoint.vi"("Error In"=w534, "Setpoint"="Setpoint", "Temp handle"=w537) -> ("Error Out"=w533:errorcluster)  [unwired: 8 in]
        n199 = call <vilib>:"Release Semaphore.vi"("error in (no error)"=w533, "semaphore"=w531) -> ("error out"=w532:errorcluster)  [unwired: 4 in, 1 out]
      }
      event "Sampling rate", "Capture duration": Value Change; User Event {
        # "Recalculate measurement time and number of samples"
        n200 = event-data() -> ()  [unwired: 1 in, 1 out]
        n201 = local read "Capture duration"() -> (w548:dbl[unit])
        n202 = local read "Sampling rate"() -> (w546:dbl)
        n203 = node(w546) -> (w545:dbl[unit])
        n204 = Multiply(x=w545, y=w548) -> (x*y=w544:dbl)
        n205 = Greater?(x=w544, y=200000.0) -> (0:w542:bool)
        n206 = property on="No samples" class="DigNum (strict)"(error in=w549, "Val(Sgnl)"=w544, "Blinking"=w542) -> (error out=w547:errorcluster)  [unwired: 1 in, 1 out]
      }
      event "2 pulse mode": Value Change {
        n207 = event-data() -> ("NewVal"=w553:bool)  [unwired: 1 in]
        n208 = Select(t=T26."Enabled" ("Disabled"), s=w553, f=T26."Disabled and Grayed Out") -> (s? t:f=w555:T26)
        n209 = property on="2nd pulse length" class="DigNum (strict)"(error in=w559, "DisabledEnum"=w555) -> (error out=w558:errorcluster)  [unwired: 1 in, 1 out]
        n210 = property on="2nd pulse voltage" class="DigNum (strict)"(error in=w558, "DisabledEnum"=w555) -> (error out=w557:errorcluster)  [unwired: 1 in, 1 out]
      }
      event "1st pulse length": Value Change {
        w571 = dbl[unit] 2.333e-07  # s
        # "Coerce length of the filling pulse to values available in MFIA"
        n211 = event-data() -> ("CtlRef"=w570:refnum<vi>, "NewVal"=w568:dbl[unit])  [unwired: 1 in]
        n212 = Divide(x=w568, y=w571) -> (x/y=w573:dbl)
        n213 = Round To Nearest(number=w573) -> (nearest integer value=w572:dbl)
        n214 = Multiply(x=w572, y=w571) -> (x*y=w569:dbl[unit])
        n215 = property class="DigNum (strict)"(reference=w570, error in=w567, "Value"=w569) -> (error out=w566:errorcluster)  [unwired: 1 out]
      }
      event "Measure": Value Change {
        w603 = FALSE ("Visible")
        w601 = T26."Disabled and Grayed Out" ("Disabled")
        # "Rename folder"
        # "New Folder"
        # "Old Folder"
        # "Send Settings and LDLTS params to MHL"
        # "Flag measurement as \"modified\""
        # "Prepare Front Panel (incl. plots) for a measurement, trigger Measurement Handling Loop"
        n216 = event-data() -> ()  [unwired: 1 in, 1 out]
        n217 = invoke on="Transient Graph" class="XYGraph (strict)" method="Reinit To Default"(error in=w577) -> (error out=w576:errorcluster)  [unwired: 2 in, 2 out]
        n218 = property on="Temperature" class="DigNum (strict)"(error in=w576) -> (error out=w595:errorcluster, "Value"=w594:dbl[unit])  [unwired: 1 in, 1 out]
        n219 = Unbundle By Name(w618) -> ("Folder"=w591:path, "LDLTS properties"=w624:T3)
        n220 = node("Sampling rate") -> (w606:dbl[unit])
        n221 = Bundle By Name(cluster=w624, "Averaging"="Averaging", "I range"="I range", "Test signal"="Test signal", "V range"="V range", "Test frequency"="Test frequency", "Vbias"="Bias voltage", "Vpulse"="1st pulse voltage", "pulse length"="1st pulse length", "Sampling time"="Capture duration", "Sampling rate"=w606, "Bandwidth"="Bandwidth", "Pulse 2"="2 pulse mode", "Vpulse 2"="2nd pulse voltage", "pulse length 2"="2nd pulse length", "Acq. delay"="Acquisition delay", "Filter order"="Filter order", "Equivalent circuit model"="Model", "T"=w594) -> (w617:T3)
        n222 = property on="Save Parameters" class="Bool (strict)"(error in=w595, "Visible"=w603) -> (error out=w602:errorcluster)  [unwired: 1 in, 1 out]
        n223 = property on="Export" class="Bool"(error in=w602, "Visible"=w603) -> (error out=w583:errorcluster)  [unwired: 1 in, 1 out]
        n224 = call "myDLTS GUID.vi"() -> ("GUID"=w581:string)  [unwired: 1 in]
        n225 = Strip Path(path=w591) -> (stripped path=w593:path)  [unwired: 1 out]
        n226 = local read "Workspace"() -> (w592:path)
        n227 = Build Path(base path=w593, name or relative path=w581) -> (appended path=w590:path)
        n228 = Build Path(base path=w592, name or relative path=w591) -> (appended path=w589:path)
        n229 = Get Date/Time In Seconds() -> (seconds since 1Jan1904=w582:timestamp)
        n230 = Build Path(base path=w592, name or relative path=w590) -> (appended path=w587:path)
        n231 = local write "Folder"(w590) -> ()
        n232 = Bundle By Name(cluster=w618, "GUID"=w581, "Folder"=w590, "Time"=w582, "LDLTS properties"=w617) -> (w616:T2)
        n233 = call <vilib>:"Check if File or Folder Exists.vi"("error in (no error)"=w583, "path"=w589) -> ("error out"=w586:errorcluster, "file or folder exists?"=w585:bool, "dup path"=w588:path)  [unwired: 7 in]
        n234 = case shown="True" w585 {
          tunnel: w588 -> [_ w636]
          tunnel: w587 -> [_ w635]
          tunnel: w586 -> [w632 w634]
          tunnel: [w632 w633] -> w584
          frame False {
          }
          frame True {
            n235 = Move(source path=w636, error in=w634, 9:TRUE ("overwrite (F)"), 10:w635) -> (error out=w633:errorcluster)  [unwired: 1 in, 2 out]
          }
        }
        n236 = Unbundle By Name(w631) -> ("Settings"=w630:T12)
        n237 = property on="Setpoint" class="DigNum (strict)"(error in=w584, "DisabledEnum"=w601) -> (error out=w600:errorcluster)  [unwired: 1 in, 1 out]
        n238 = Bundle By Name(cluster=cluster{"Settings":T12, "LDLTS properties":T3} {"Settings"={"MFIA"={"Address"="", "Use compensation"=TRUE, "Shut down gracefully"=FALSE}, "Temp ctrl"={"Gain (P)"=0.0, "Reset (I)"=0.0, "Rate (D)"=0.0, "Stabilization rate"=0.0, "Stabilization delta"=0.0, "Type"=enum."Lake Shore 325", "Custom temp ctrl"={"VISA resource name"=""}, "Lakeshore 325"={"VISA name"="", "Loop"=0, "Heater Range"=1, "Heater Resistance"=0, "Sample sensor"=0, "Fast sensor"=0, "Slow sensor"=0}, "Lakeshore 331"={"VISA name"="", "Loop"=1, "Heater Range"=0, "Sample sensor"=0, "Fast sensor"=0, "Slow sensor"=0}, "Lakeshore 332"={"VISA name"="", "Loop"=1, "Heater Range"=0, "Sample sensor"=0, "Fast sensor"=0, "Slow sensor"=0}, "Lakeshore 335"={"VISA name"="", "Loop"=1, "Sample sensor"=0, "Fast sensor"=0, "Slow sensor"=0, "Heater Range"=0, "Output mode"=enum."Off"}, "Lakeshore 336"={"VISA name"="", "Loop"=1, "Output mode"=enum."Off", "Max current"=1.0, "Heater resistance"=1, "Sample sensor"=1, "Slow sensor"=1, "Fast sensor"=1}}, "Source-meter"={"Type"=enum."Custom", "Custom source-meter"={"VISA resource name"=""}, "Keithley 2600"={"VISA name"="", "Ignore ID Query"=FALSE, "SMU"=enum."Channel A"}, "Keithley 2400 Series"={"VISA name"="", "Ignore ID Query"=FALSE}}, "Other"={"Enable OriginLab"=FALSE, "Reader mode"=FALSE, "Auto-save"=FALSE}, "Defaults"={"IV properties"={"T"=0.0, "Vstart"=-0.5, "Vstop"=0.5, "Vpoints"=10.0, "Settling"=0.01, "I limit"=0.1, "Log mapping"=FALSE, "Averaging"=0.0}, "CV properties"={"T"=0.0, "Vstart"=-0.5, "Vstop"=0.5, "Vpoints"=10.0, "Precision"=enum."Normal", "Test signal"=0.01, "Auto I range"=FALSE, "Test frequency"=100000.0, "I range"=-2.0, "V range"=10.0, "Log mapping"=FALSE, "Rel perm"=0.0, "Area"=0.0, "Equivalent circuit model"=0}, "DLTS properties"={"Tstart"=0.0, "Instant start"=FALSE, "Tstop"=0.0, "T rate"=0.0, "Test signal"=0.0, "Test frequency"=0.0, "Bandwidth"=0.0, "Averaging"=0.0, "Vbias"=0.0, "Vpulse"=0.0, "pulse length"=0.0, "Pulse 2"=FALSE, "Vpulse 2"=0.0, "pulse length 2"=0.0, "I range"=-2.0, "V range"=10.0, "Emission rate"=[], "Sampling rate"=0.0, "Acq. delay"=0.0, "Filter order"=0, "Equivalent circuit model"=0}, "LDLTS properties"={"T"=0.0, "Test signal"=0.0, "Test frequency"=0.0, "Bandwidth"=0.0, "Averaging"=0.0, "Vbias"=0.0, "Vpulse"=0.0, "pulse length"=0.0, "Pulse 2"=FALSE, "Vpulse 2"=0.0, "pulse length 2"=0.0, "I range"=-2.0, "V range"=10.0, "Sampling rate"=0.0, "Acq. delay"=0.0, "Sampling time"=0.0, "Filter order"=0, "Equivalent circuit model"=0}}}, "LDLTS properties"={"T"=0.0, "Test signal"=0.0, "Test frequency"=0.0, "Bandwidth"=0.0, "Averaging"=0.0, "Vbias"=0.0, "Vpulse"=0.0, "pulse length"=0.0, "Pulse 2"=FALSE, "Vpulse 2"=0.0, "pulse length 2"=0.0, "I range"=-2.0, "V range"=10.0, "Sampling rate"=0.0, "Acq. delay"=0.0, "Sampling time"=0.0, "Filter order"=0, "Equivalent circuit model"=0}}, "Settings"=w630, "LDLTS properties"=w617) -> (w626:cluster{"Settings":T12, "LDLTS properties":T3})
        n239 = property on="Measure" class="Bool"(error in=w600, "DisabledEnum"=w601) -> (error out=w580:errorcluster)  [unwired: 1 in, 1 out]
        n240 = property on="Stop" class="Bool"(error in=w580, "DisabledEnum"=T26."Enabled" ("Disabled")) -> (error out=w579:errorcluster)  [unwired: 1 in, 1 out]
        n241 = Bundle By Name(cluster=cluster{"Data":variant, "Message":string} {"Data"=variant, "Message"=""}, "Data"=w626, "Message"="Prepare") -> (w628:cluster{"Data":variant, "Message":string})
        n242 = property on="Measurement info" class="Str"(error in=w579, "Value"="Initializing measurement" ("Measurement info")) -> (error out=w613:errorcluster)  [unwired: 1 in, 1 out]
        n243 = Enqueue Element(queue=w625, element=w628, error in (no error)=w613) -> (error out=w627:errorcluster)  [unwired: 1 in, 2 out]
      }
      event "Filter order", "Bandwidth": Value Change {
        n244 = event-data() -> ()  [unwired: 1 in, 1 out]
        n245 = local read "Bandwidth"() -> (w639:dbl[unit])
        n246 = local read "Filter order"() -> (w638:i32)
        n247 = call "MFIA Filter Response Calculation.vi"("Filter order"=w638, "Bandwidth"=w639) -> ("Settling times"=w641:T32)  [unwired: 8 in, 1 out]
        n248 = Unbundle By Name(w641) -> ("T_s 95%"=→"Filter rise time":dbl[unit])
      }
      event "Stop": Value Change {
        n249 = event-data() -> ()  [unwired: 1 in, 1 out]
        n250 = Set Occurrence(w646) -> ()
      }
      event "V range", "Test signal", "Bias voltage", "1st pulse voltage", "2nd pulse voltage": Value Change {
        # "Coerce voltages"
        n251 = event-data() -> ()  [unwired: 1 in, 1 out]
        n252 = property on="Test signal" class="DigNum (strict)"(error in=w652) -> (error out=w659:errorcluster, "Value"=w663:dbl[unit])  [unwired: 1 in, 1 out]
        n253 = Multiply(x=w663, y=1.42) -> (x*y=w660:dbl[unit])
        n254 = property on="V range" class="Ring (strict)"(error in=w659) -> (error out=w658:errorcluster, "Value"=w661:dbl[unit])  [unwired: 1 in, 1 out]
        n255 = control-ref of="Bias voltage"() -> (w656:refnum<vi>)
        n256 = control-ref of="1st pulse voltage"() -> (w655:refnum<vi>)
        n257 = control-ref of="2nd pulse voltage"() -> (w651:refnum<vi>)
        n258 = Subtract(x=w661, y=w660) -> (x-y=w657:dbl[unit])
        n259 = Build Array(w656, w655, w651) -> (w654:refnum<vi>[])
        n260 = for {
          tunnel: w658 -> [w671]
          tunnel: w657 -> [w670]
          tunnel: w654 -> [w668] mode=indexing
          tunnel: [w667] -> w653
          n261 = property on="Property Node" class="DigNum (strict)"(reference=w668, error in=w671) -> (reference out=w669:refnum<vi>, error out=w673:errorcluster, "Value"=w672:dbl[unit])
          n262 = Negate(x=w670) -> (-x=w676:dbl[unit])
          n263 = In Range and Coerce(upper limit=w670, x=w672, lower limit=w676) -> (coerced(x)=w674:dbl[unit], In Range?=w675:bool)
          n264 = case shown="False" w675 {
            tunnel: w674 -> [w679 _]
            tunnel: w673 -> [w680 w681]
            tunnel: [w678 w681] -> w667
            tunnel: w669 -> [w677 _]
            frame False {
              # "Coerce"
              n265 = property on="Property Node" class="DigNum (strict)"(reference=w677, error in=w680, "Value"=w679) -> (error out=w678:errorcluster)  [unwired: 1 out]
            }
            frame True {
              # "In Range"
            }
          }
        }
      }
      event "Top Buttons.Save Parameters": Value Change {
        # "Save parameters without triggering the measurement"
        n266 = event-data() -> ("NewVal"=w683:bool)  [unwired: 1 in]
        n267 = case shown="True" w683 {
          tunnel: w688 -> [w692 w715]
          tunnel: [w692 w713] -> w687
          tunnel: [w691 TRUE] -> w686
          tunnel: w685 -> [w690 w710]
          tunnel: [w690 w697] -> w684
          tunnel: w682 -> [w691 _]
          frame False {
          }
          frame True {
            n268 = Unbundle By Name(w715) -> ("LDLTS properties"=w716:T3)
            n269 = local read "Acquisition delay"() -> (w709:dbl[unit])
            n270 = local read "2 pulse mode"() -> (w708:bool)
            n271 = local read "Bandwidth"() -> (w698:dbl[unit])
            n272 = local read "Averaging"() -> (w699:dbl)
            n273 = local read "I range"() -> (w700:dbl)
            n274 = local read "Test signal"() -> (w701:dbl[unit])
            n275 = local read "V range"() -> (w702:dbl[unit])
            n276 = local read "Test frequency"() -> (w703:dbl[unit])
            n277 = local read "Bias voltage"() -> (w704:dbl[unit])
            n278 = local read "1st pulse voltage"() -> (w705:dbl[unit])
            n279 = local read "1st pulse length"() -> (w706:dbl[unit])
            n280 = local read "Capture duration"() -> (w707:dbl[unit])
            n281 = local read "Sampling rate"() -> (w696:dbl)
            n282 = local read "2nd pulse voltage"() -> (w693:dbl[unit])
            n283 = local read "2nd pulse length"() -> (w694:dbl[unit])
            n284 = node(w696) -> (w695:dbl[unit])
            n285 = Bundle By Name(cluster=w716, "Acq. delay"=w709, "Pulse 2"=w708, "Bandwidth"=w698, "Averaging"=w699, "I range"=w700, "Test signal"=w701, "V range"=w702, "Test frequency"=w703, "Vbias"=w704, "Vpulse"=w705, "pulse length"=w706, "Sampling time"=w707, "Sampling rate"=w695, "Vpulse 2"=w693, "pulse length 2"=w694) -> (w714:T3)
            n286 = property on="Measurement info" class="Str"(error in=w710, "Value"="Parameters saved" ("Measurement info")) -> (error out=w697:errorcluster)  [unwired: 1 in, 1 out]
            n287 = Bundle By Name(cluster=w715, "LDLTS properties"=w714) -> (w713:T2)
          }
        }
      }
      event "Top Buttons.Information": Value Change {
        # "Display Info dialog"
        n288 = event-data() -> ("NewVal"=w723:bool)  [unwired: 1 in]
        n289 = case shown="True" w723 {
          tunnel: w722 -> [w726 w733]
          tunnel: w718 -> [w725 w736]
          tunnel: [w725 w734] -> w717
          tunnel: [w726 w732] -> w721
          tunnel: w719 -> [w727 w731]
          tunnel: [w727 w730] -> w720
          frame False {
          }
          frame True {
            n290 = Unbundle By Name(w733) -> ("Name"=w738:string, "Comment"=w737:string)
            n291 = call "Measurement renamer.vi"("error in (no error)"=w736, "Comment In"=w737, "Measurement name In"=w738) -> ("error out"=w734:errorcluster, "Canceled"=w735:bool, "Comment Out"=w728:string, "Measurement name Out"=w729:string)  [unwired: 1 in]
            n292 = case shown="False" w735 {
              tunnel: w733 -> [w742 w745]
              tunnel: [w741 w745] -> w732
              tunnel: w731 -> [_ w744]
              tunnel: [TRUE w744] -> w730
              tunnel: w729 -> [w740 _]
              tunnel: w728 -> [w739 _]
              frame False {
                n293 = Bundle By Name(cluster=w742, "Name"=w740, "Comment"=w739) -> (w741:T2)
              }
              frame True {
              }
            }
          }
        }
      }
      event "Top Buttons.Export": Value Change {
        # "Display Export dialog and export data"
        n294 = event-data() -> ()  [unwired: 1 in, 1 out]
        n295 = Unbundle By Name(w751) -> ("Settings.Other.Enable OriginLab"=w750:bool)
        n296 = Bundle By Name(cluster=T31 {"Clipboard"=TRUE, "dat"=TRUE, "iso"=FALSE, "Origin"=FALSE, "Excel"=FALSE} ("Available options"), "Origin"=w750) -> (w752:T31)
        n297 = local read "Workspace"() -> (w754:path)
        n298 = call "Export dialog.vi"("error in (no error)"=w753, "Available options"=w752) -> ("error out"=w749:errorcluster, "Option"=w748:T33)  [unwired: 7 in, 1 out]
        n299 = case shown="\"Dat\"" w748 {
          tunnel: w749 -> [w759 w762 w768 w773]
          tunnel: [w759 w760 w767 w772] -> w757
          tunnel: w756 -> [_ w761 w766 w771]
          tunnel: w755 -> [_ _ _ w770]
          tunnel: w754 -> [_ w763 w765 w769]
          tunnel: "myDLTS file path" -> [_ _ w764 _]
          frame "Canceled", Default {
          }
          frame "Clipboard" {
            n300 = call-poly "Export single clipboard - cluster.vi"("Error In"=w762, "Workspace"=w763, "LDLTS measurement"=w761) -> ("Error Out"=w760:errorcluster)  [unwired: 5 in]
          }
          frame "Dat" {
            n301 = call-poly "Export single dat - cluster.vi"(".myDLTS file path"=w764, "Error In"=w768, "Workspace"=w765, "LDLTS measurement"=w766) -> ("Error Out"=w767:errorcluster)  [unwired: 4 in]
          }
          frame "Origin" {
            n302 = call-poly "Export Origin.vi"("Error In"=w773, "Workspace"=w769, "Session properties"=w770, "LDLTS measurement"=w771) -> ("Error Out"=w772:errorcluster)  [unwired: 7 in]
          }
        }
      }
    }
    n303 = call <vilib>:"General Error Handler.vi"("type of dialog (OK msg:1)"=w452, "error in (no error)"=w453) -> ("error out"=w454:errorcluster)  [unwired: 9 in, 4 out]
    n304 = call <vilib>:"Clear Errors.vi"("error in (no error)"=w454) -> ("error out"=w450:errorcluster)  [unwired: 5 in, 1 out]
  }
  "Loop data out" <- w113
  "Modified" <- w84
  "LDLTS measurement out" <- w35
  n305 = Unregister For Events(event registration refnum=w90, error in=w91) -> (error out=w39:errorcluster)
  n306 = Destroy User Event(user event=w37, error in=w39) -> (error out=w38:errorcluster)
  n307 = Destroy User Event(user event=w49, error in=w38) -> (error out=w79:errorcluster)
  n308 = Merge Errors(w79, w77) -> (w78:errorcluster)
  n309 = Release Queue(queue=w89, error in (no error)=w78) -> (error out=→"Error Out":errorcluster)  [unwired: 1 in, 2 out]
